vi "FileExplorerMain.vi"(0 "Top Level Folder Path":path, 4 "Tree":string[](tree), 5 "Search Bar":string, 7 "Copy":bool, 9 "Expand / Colapse":bool, 11 "error in (no error)":errorcluster) -> (6 "Report String":string, 15 "error out":errorcluster)   [LabVIEW 2023]
doc: "This VI is the demonstration of the File explorer using tree with options like search, copy, expand/collapse the tree items populated from the input file path."
uses:
  TypeDefs/FileExplorerQueueOperations.ctl
  TypeDefs/FileExplorerStateDataCluster.ctl
  TypeDefs/FileExplorerDataCluster.ctl
  TypeDefs/ReportDetailsCluster.ctl
  TypeDefs/TreeSortCluster.ctl
  TypeDefs/FilesandFoldersPath.ctl
  TypeDefs/FileSelectionCluster.ctl
  TypeDefs/TagsCluster.ctl
panel:
  # "INSTRUCTIONS\n\n1. Run the VI.\n2. Choose the any folder path using \"Top Level Folder Path\" Control.\n3. Tree is populated with the selected folder hierarchy.\n4. Press \"Expand/Collapse\" button to expand or collapse the Folders in the tree.\n5. Enter folder name in the \"Search Bar\" and press enter to expand on particular folder.\n6. Select any files in the tree and press \"Copy\" to copy the file to the desired location.\n7. Whenever a folder is expanded, particular folder details is indicated in the \"Report String\"\n8. Press the Column Headers to sort the tree based on the selection like Date Modified, Type or size"
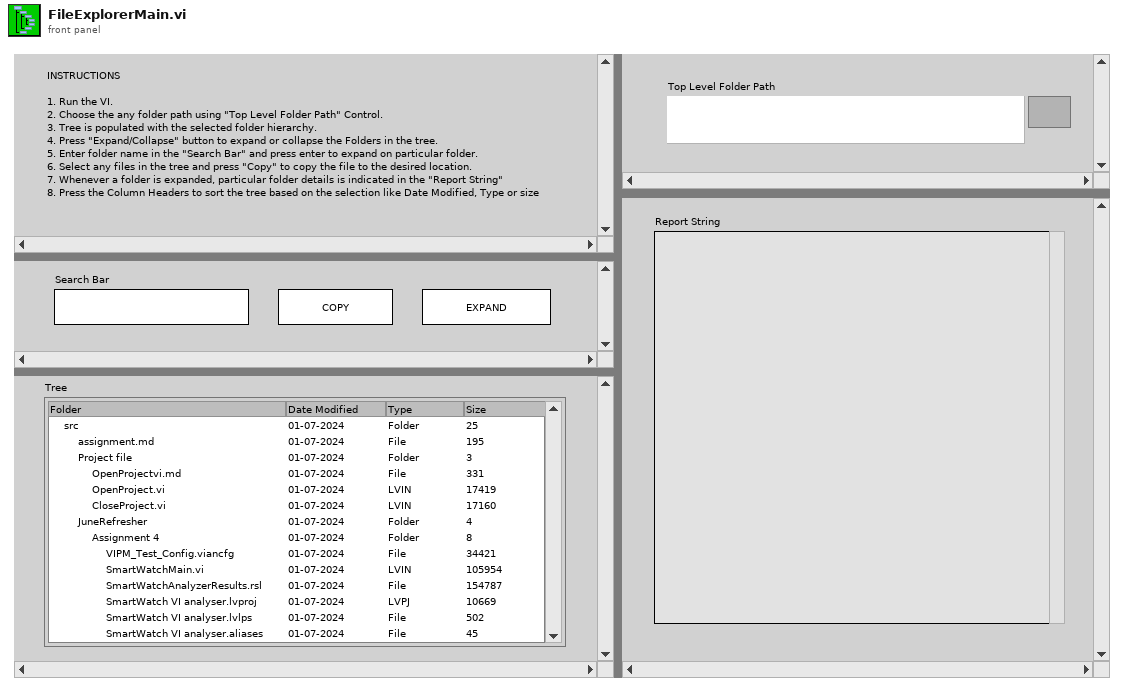
[diagram p1: front panel]
types:
  T1 = typedef "FileExplorerDataCluster.ctl" = cluster{"user event ref":refnum<user-event>, "Search Bar":string, "Tag Path":string[], "Copied File Path array":path[], "Copy file Folder":string, "Folders Array":string[], "Report details":T2, "Sort Flag":T3, "Paths":T4, "File Selection":T5, "Tags":T6, "TagSymbol Array":string[], "Path Tag":string, "New Folder Tag":path, "New Folder":bool, "Folder Found":bool, "Searched Folder Tag":string[]}
  T2 = typedef "ReportDetailsCluster.ctl" = cluster{"Tag Date Modified":string, "Tag Size":string, "Tag Type":string, "Report String":string}
  T3 = typedef "TreeSortCluster.ctl" = cluster{"Sort Date":bool, "Sort Type":bool, "Sort Size":bool}
  T4 = typedef "FilesandFoldersPath.ctl" = cluster{"File Path":path, "All Folders Path":path[], "All Files Path":path[], "Temp File Path":path, "New Folder Dialog":path}
  T5 = typedef "FileSelectionCluster.ctl" = cluster{"Files Selected ?":bool, "Selected file array":string[], "First Selection":string}
  T6 = typedef "TagsCluster.ctl" = cluster{"Parent Tag":string, "Active Tag":string}
  T7 = typedef "FileExplorerStateDataCluster.ctl" = cluster{"State":string, "Data":variant}
  T8 = typedef "FileExplorerQueueOperations.ctl" = enum16{"Init", "Enqueue", "Dequeue", "Enqueue N", "Flush", "Close", "Enqueue N Stack"}
  T9 = typedef "LVPoint32TypeDef.ctl" = cluster{"Horizontal":i32, "Vertical":i32}
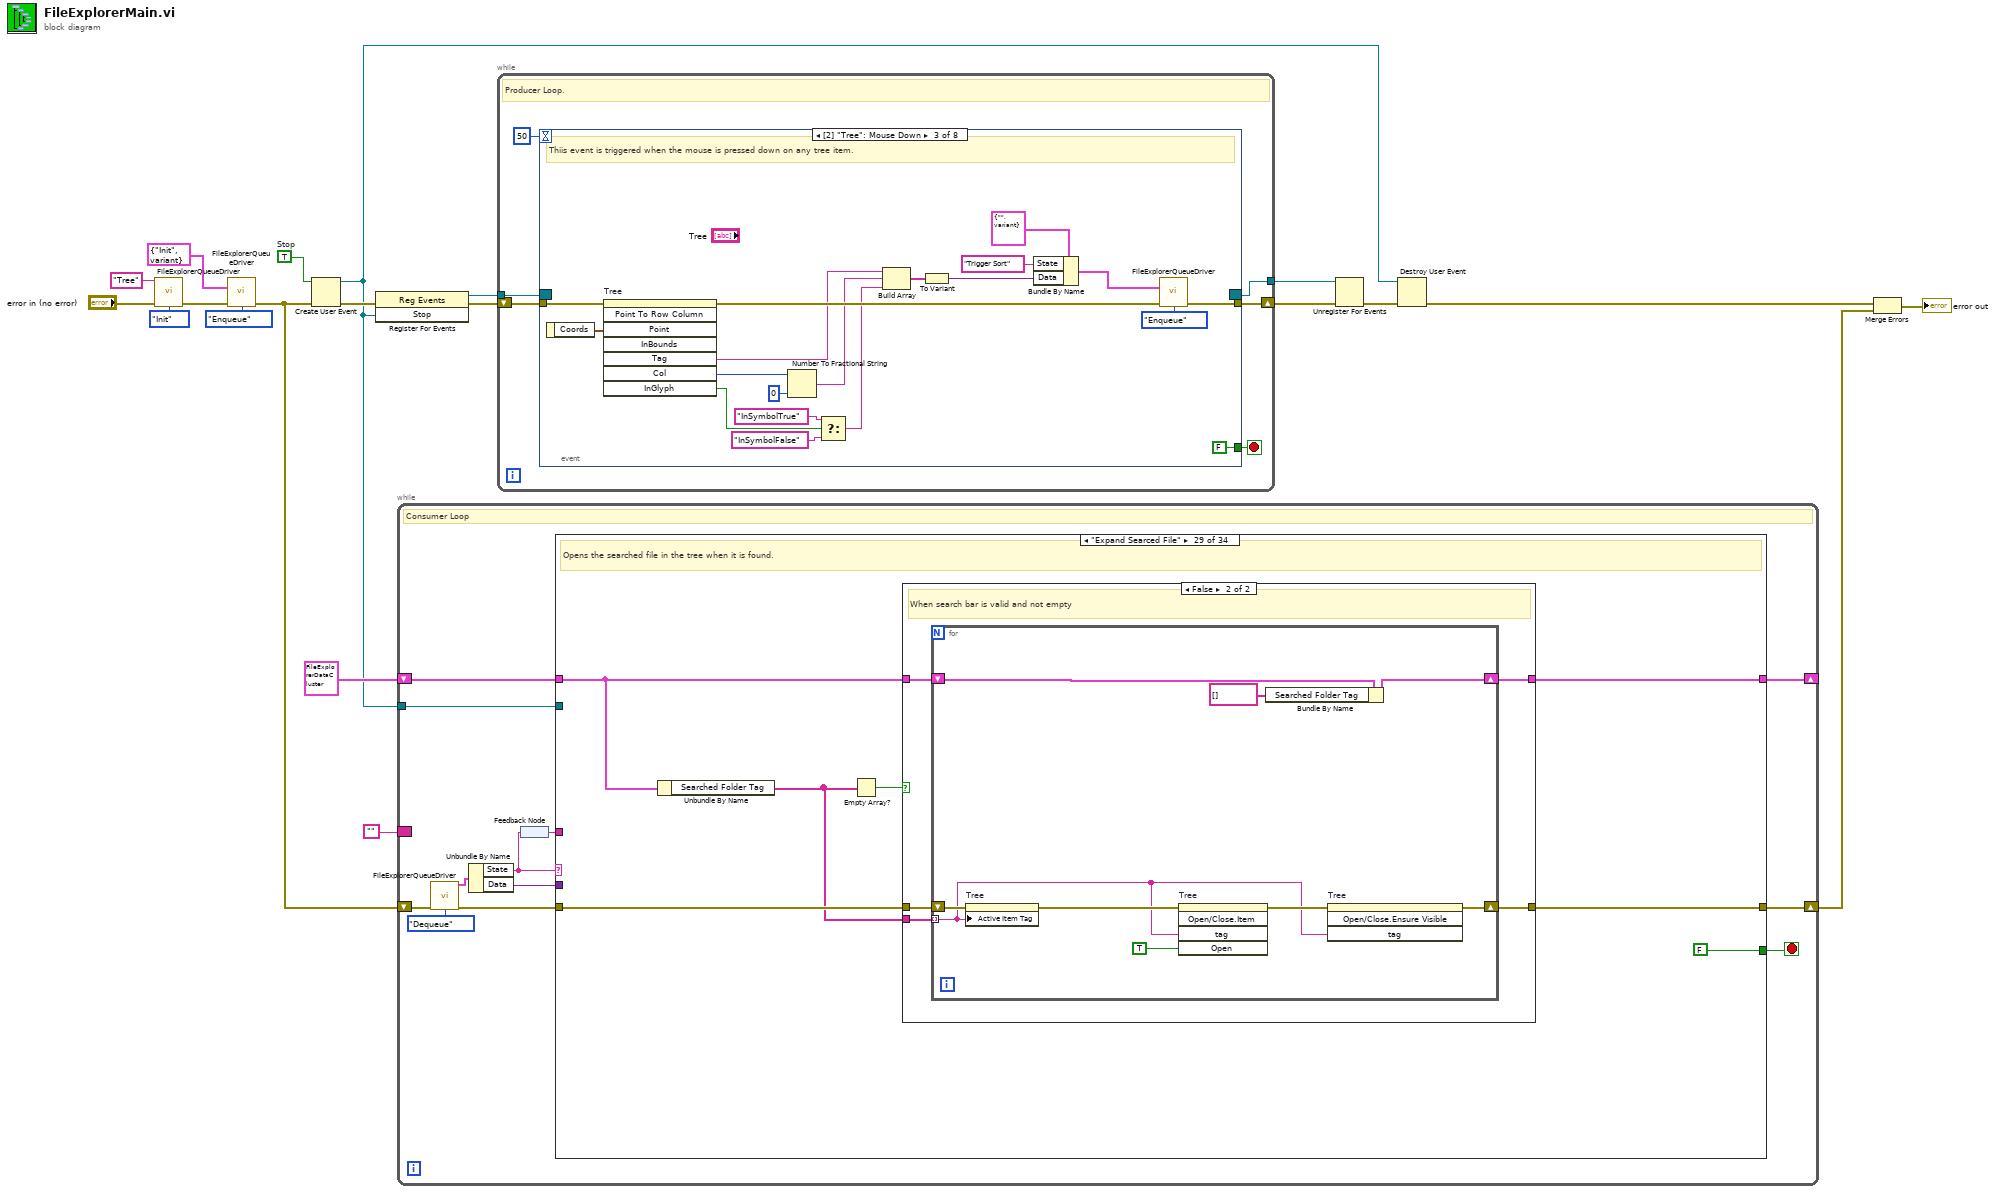
[diagram p0: block diagram]
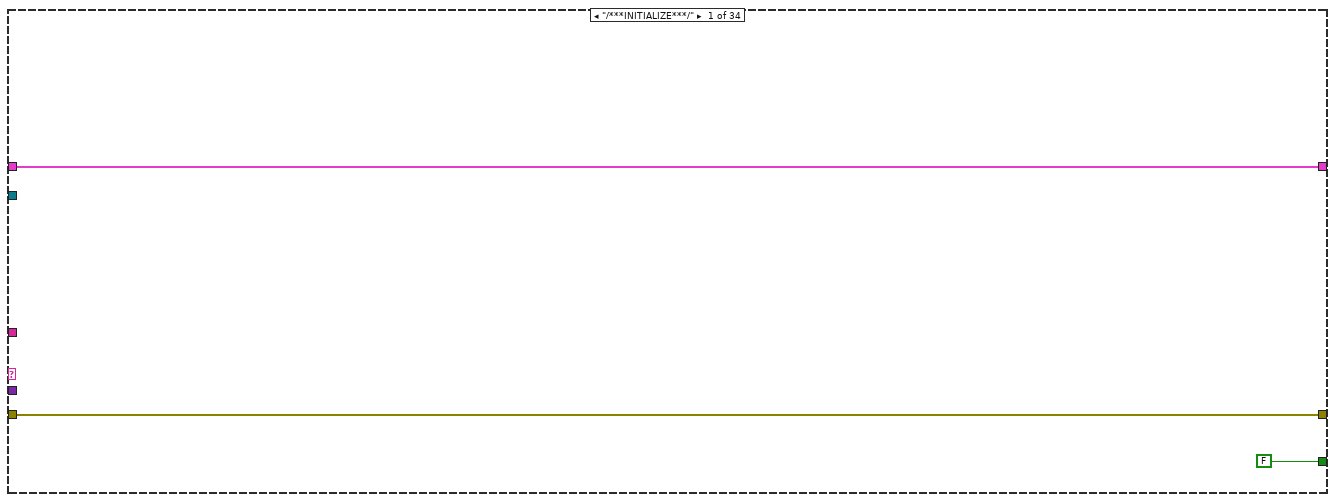
[diagram p2: hidden frame]
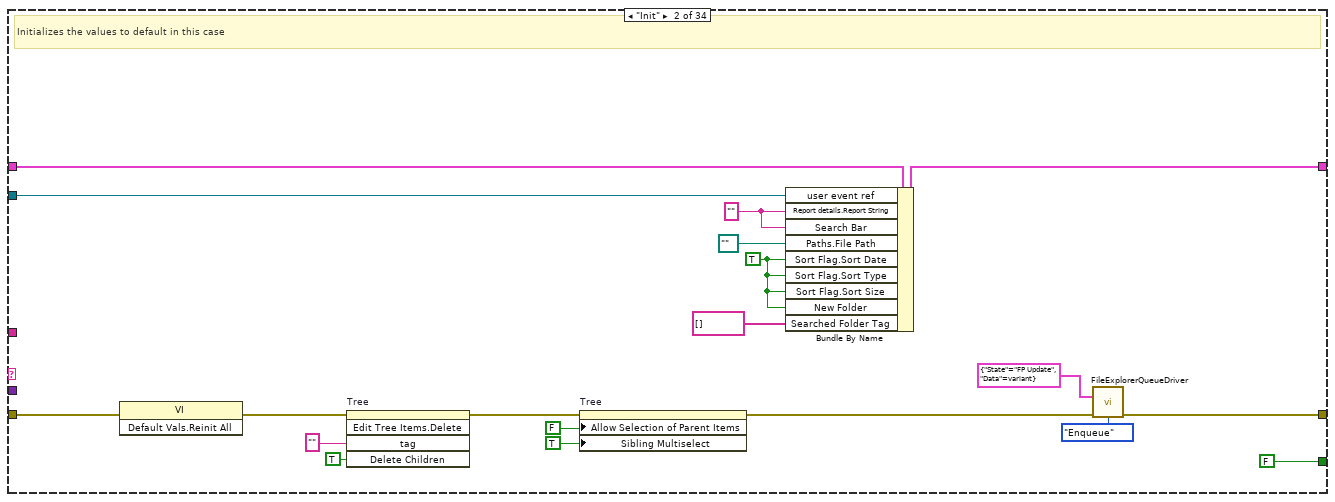
[diagram p3: hidden frame]
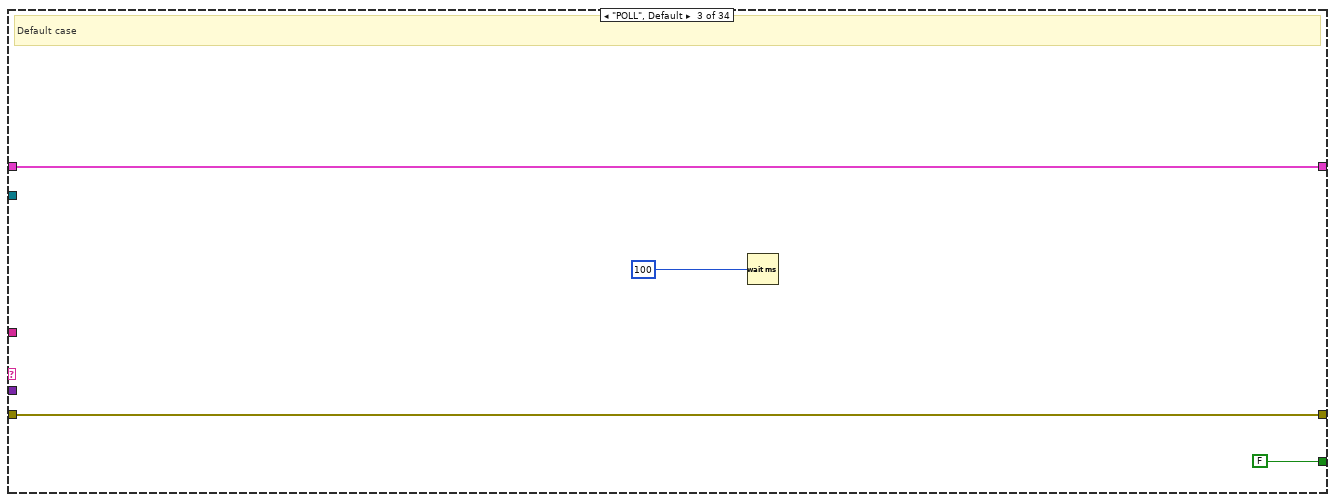
[diagram p4: hidden frame]
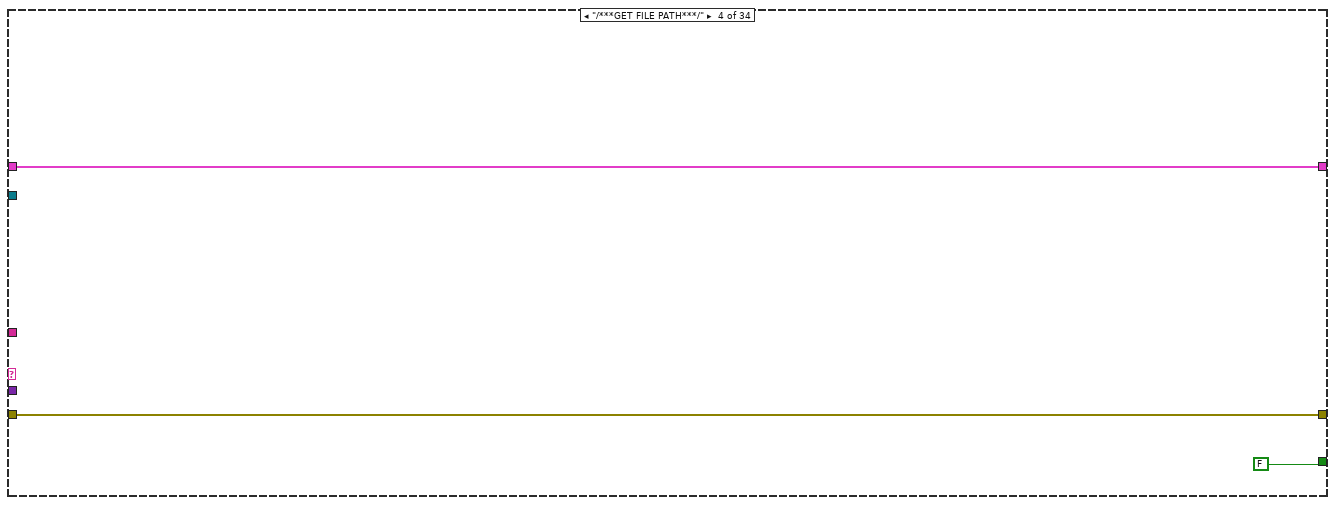
[diagram p5: hidden frame]
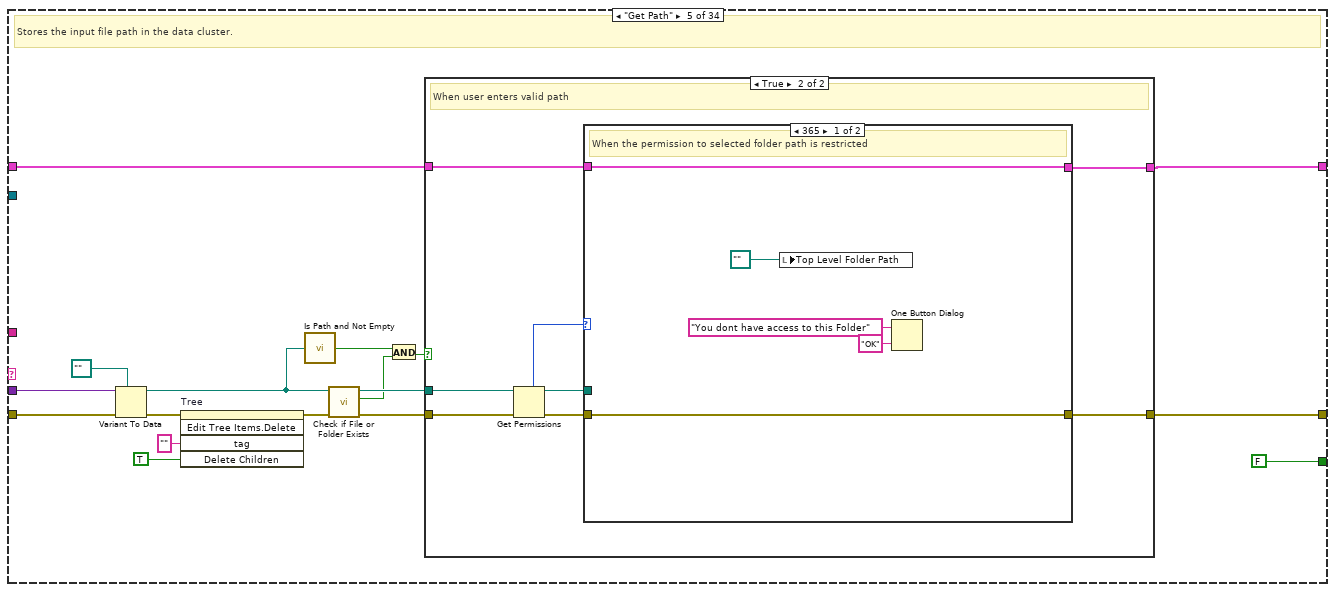
[diagram p6: hidden frame]
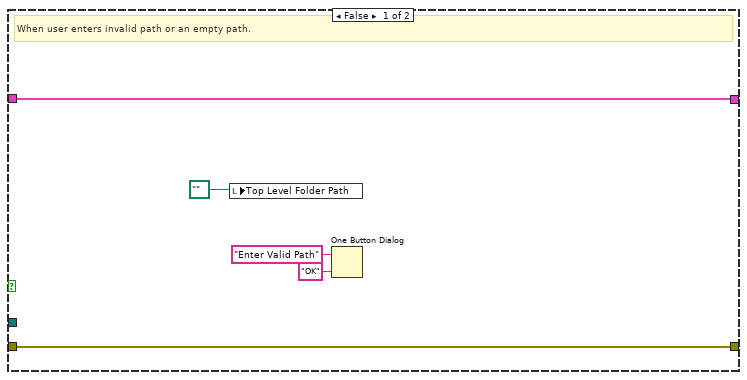
[diagram p7: hidden frame]
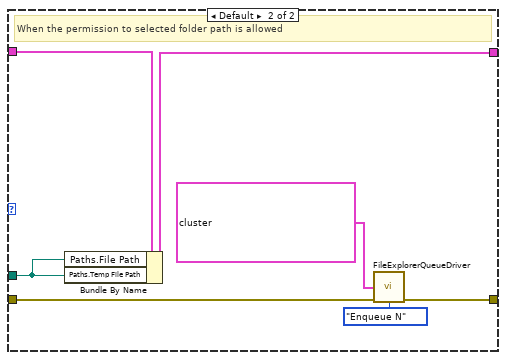
[diagram p8: hidden frame]
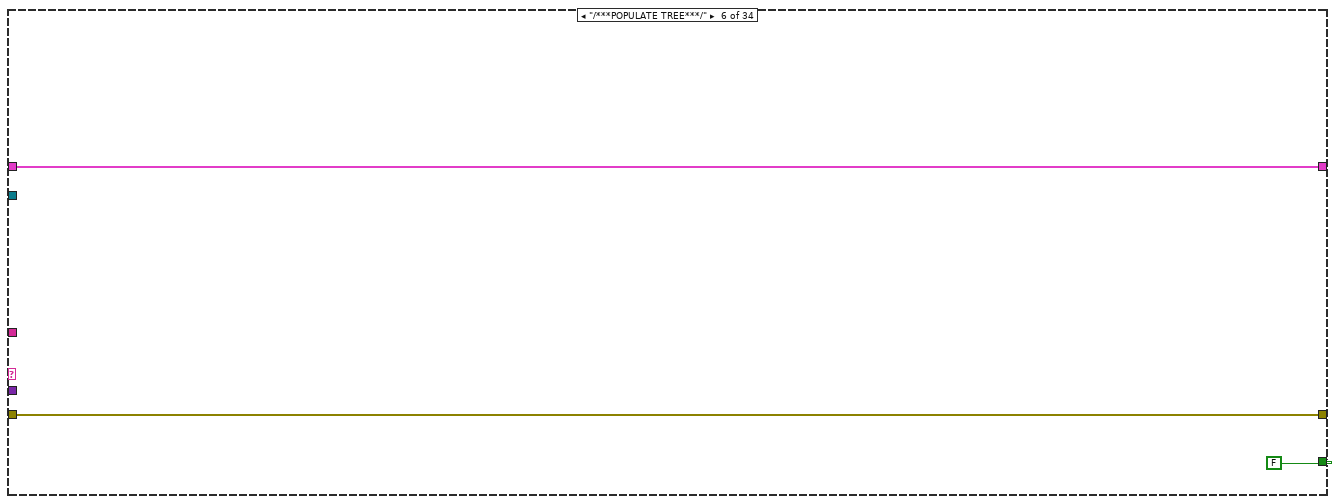
[diagram p9: hidden frame]
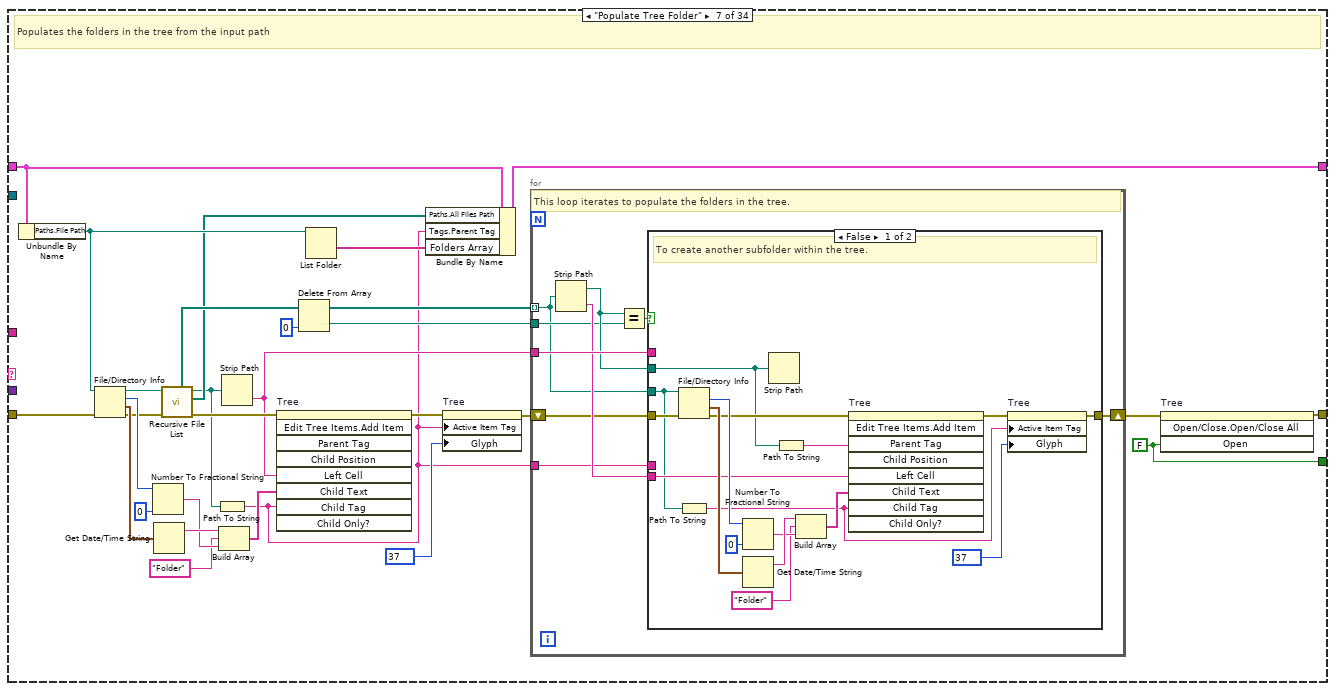
[diagram p10: hidden frame]
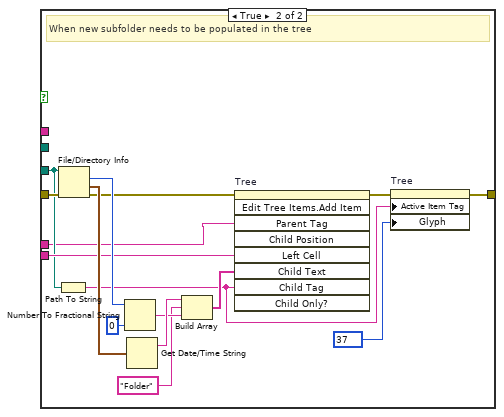
[diagram p11: hidden frame]
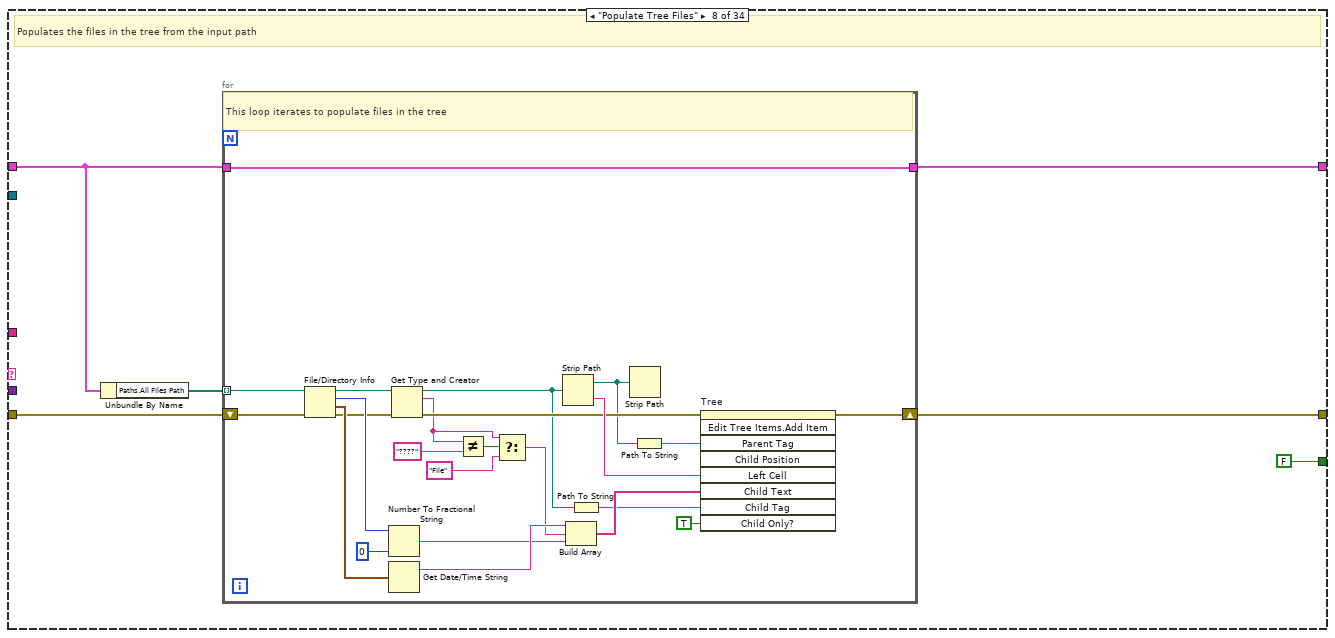
[diagram p12: hidden frame]
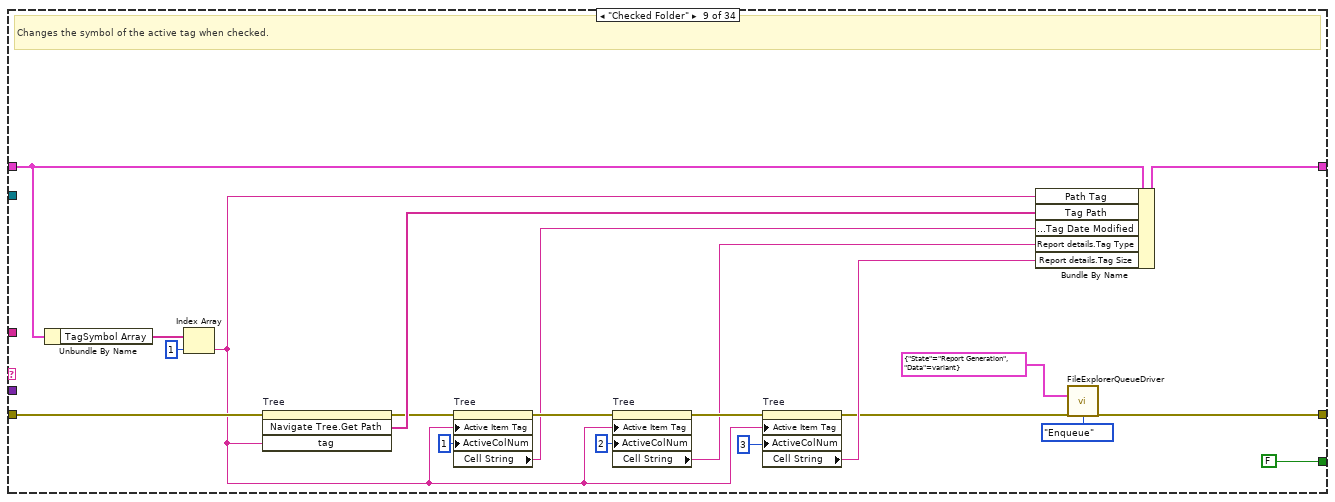
[diagram p13: hidden frame]
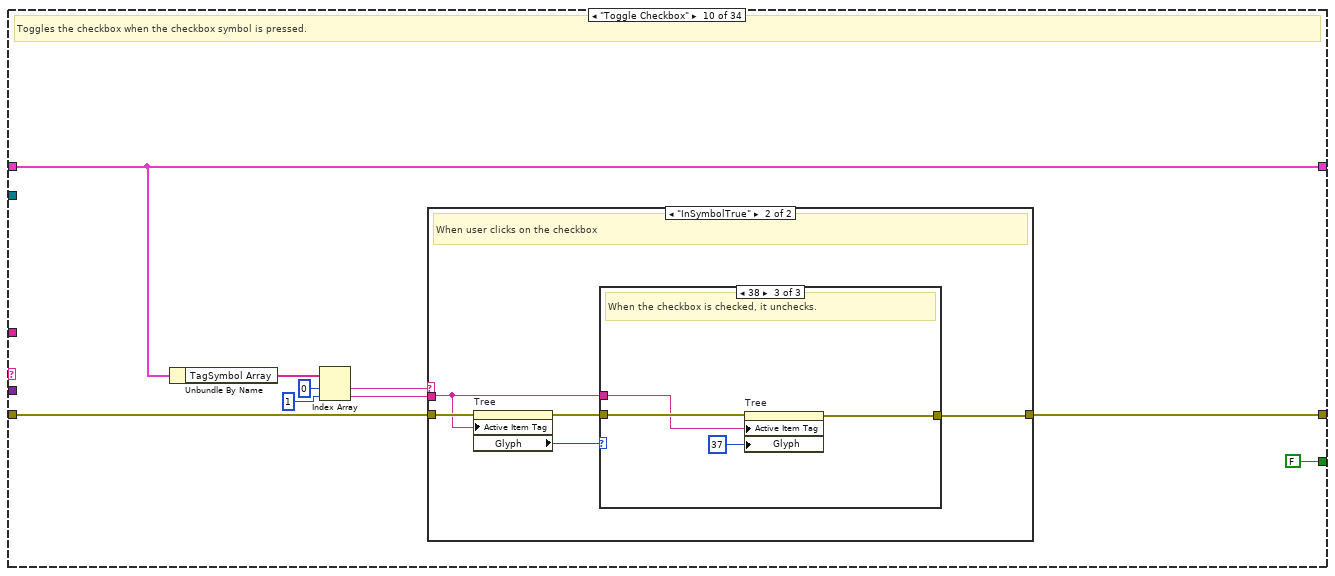
[diagram p14: hidden frame]
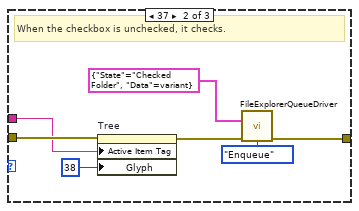
[diagram p17: hidden frame]
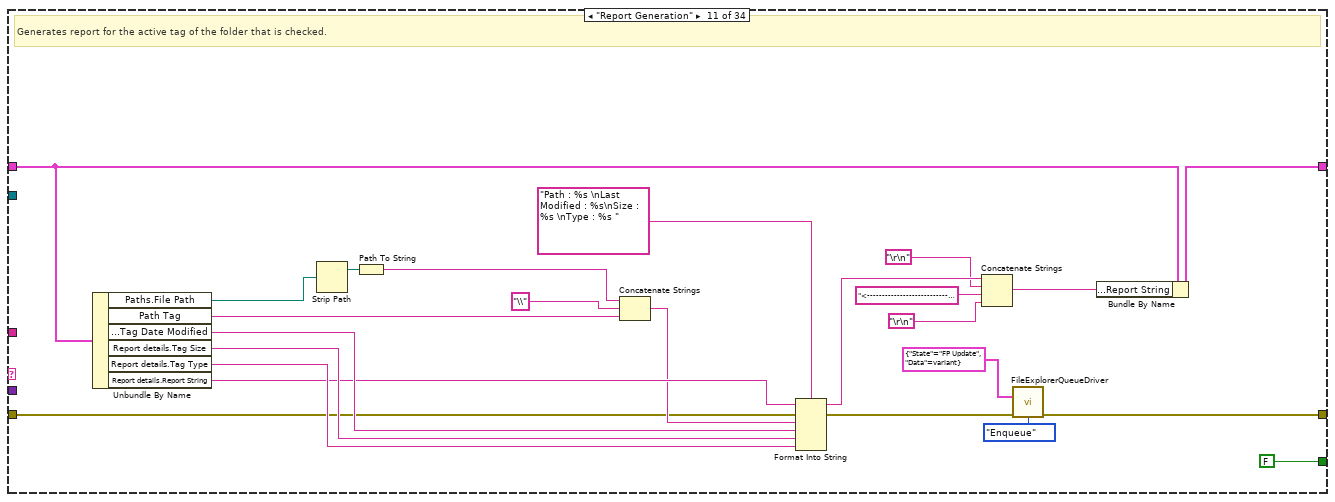
[diagram p18: hidden frame]
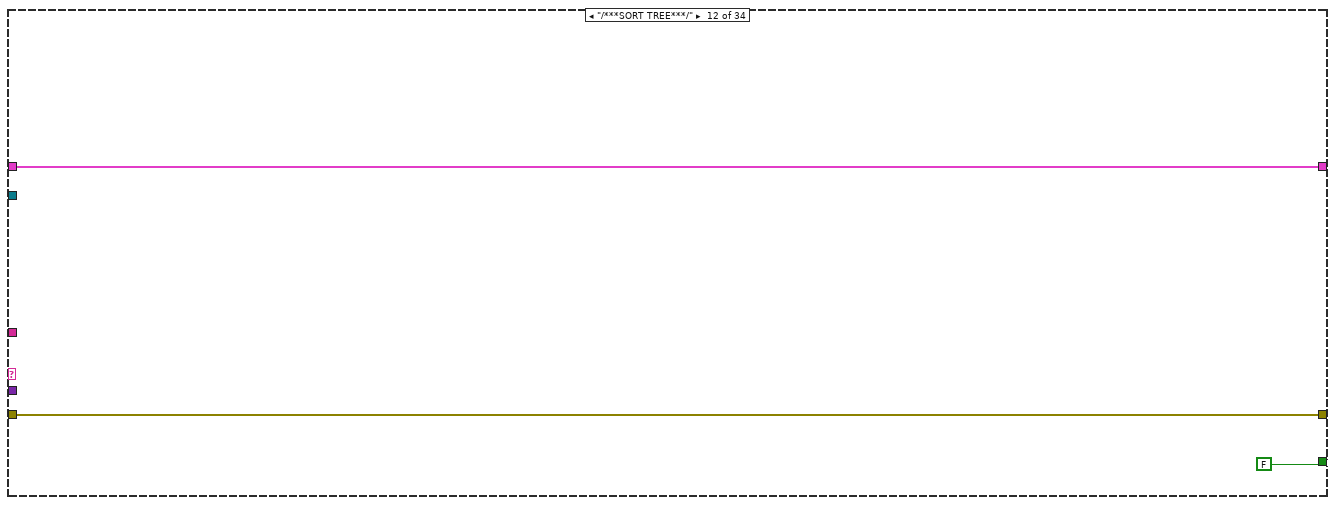
[diagram p19: hidden frame]
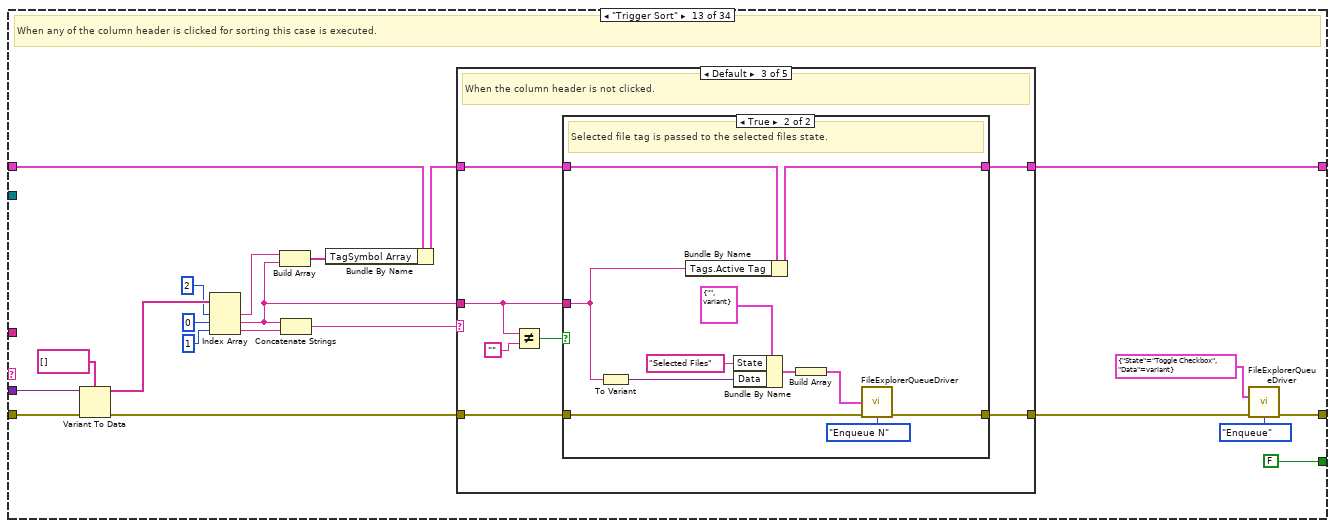
[diagram p20: hidden frame]
diagram:
  w10 = TRUE  # Stop
  n1 = call "FileExplorerQueueDriver.vi"("Queue Name"="Tree", "error in (no error)"="error in (no error)", "Enum"=FileExplorerQueueOperations."Init") -> ("error out"=w13:errorcluster)  [unwired: 11 in, 1 out]
  n2 = call "FileExplorerQueueDriver.vi"("Enqueue Element"=T7 {"State"="Init", "Data"=variant}, "error in (no error)"=w13, "Enum"=FileExplorerQueueOperations."Enqueue") -> ("error out"=w2:errorcluster)  [unwired: 11 in, 1 out]
  n3 = Create User Event(user event datatype=w10, error in=w2) -> (user event=w3:refnum<user-event>, error out=w11:errorcluster)
  n4 = register-events(error in=w11, w3) -> (reference out=w8:refnum<event-registration>, error out=w9:errorcluster)  [unwired: 1 in]
  n5 = while {
    shift-right: [w30] -> w17
    shift-left: w2 -> [w32]
    tunnel: w3 -> [w25]
    shift-right: [w23] -> _
    shift-left: T1 {"user event ref"=refnum, "Search Bar"="", "Tag Path"=[], "Copied File Path array"=[], "Copy file Folder"="", "Folders Array"=[], "Report details"={"Tag Date Modified"="", "Tag Size"="", "Tag Type"="", "Report String"=""}, "Sort Flag"={"Sort Date"=FALSE, "Sort Type"=FALSE, "Sort Size"=FALSE}, "Paths"={"File Path"=path "", "All Folders Path"=[], "All Files Path"=[], "Temp File Path"=path "", "New Folder Dialog"=path ""}, "File Selection"={"Files Selected ?"=FALSE, "Selected file array"=[], "First Selection"=""}, "Tags"={"Parent Tag"="", "Active Tag"=""}, "TagSymbol Array"=[], "Path Tag"="", "New Folder Tag"=path "", "New Folder"=FALSE, "Folder Found"=FALSE, "Searched Folder Tag"=[]} -> [w24]
    border: "" ("State") -> [_]
    stop <- w28 stop-if-true
    # "Consumer Loop"
    n6 = call "FileExplorerQueueDriver.vi"("error in (no error)"=w32, "Enum"=FileExplorerQueueOperations."Dequeue") -> ("Dequeue Element"=w27:T7, "error out"=w31:errorcluster)  [unwired: 12 in]
    n7 = Unbundle By Name(w27) -> ("State"=w22:string, "Data"=w26:variant)
    n8 = feedback #1() -> (w21:string)
    n9 = feedback-in #1(w22) -> ()
    n10 = case shown="\"Expand Searced File\"" w22 {
      tunnel: w31 -> [w34 w48 w58 w60 w76 w105 w114 w181 w212 w232 w257 w281 w303 w350 w380 w415 w426 w432 w458 w463 w513 w540 w590 w628 w678 w690 w700 w715 w736 w760 w765 w767 w780 w801]
      tunnel: [w34 w45 w58 w60 w70 w105 w121 w180 w216 w231 w267 w281 w284 w346 w376 w414 w425 w428 w458 w464 w515 w543 w584 w636 w678 w685 w700 w702 w737 w760 w765 w767 w786 w799] -> w30
      tunnel: [FALSE FALSE FALSE FALSE FALSE FALSE w115 FALSE FALSE FALSE ("Open?") FALSE FALSE FALSE FALSE FALSE FALSE FALSE FALSE FALSE FALSE FALSE ("Open?") FALSE ("Open?") FALSE FALSE FALSE FALSE FALSE FALSE FALSE FALSE FALSE FALSE FALSE TRUE] -> w28
      tunnel: w26 -> [_ _ _ _ w75 _ _ _ _ _ _ _ w302 _ _ w407 w418 _ _ _ _ _ w589 _ _ w688 _ w714 _ _ _ _ _ _]
      tunnel: w25 -> [_ w51 _ _ _ _ _ _ _ _ _ _ _ _ _ _ _ _ _ _ _ _ _ _ _ _ _ _ _ _ _ _ _ _]
      tunnel: w24 -> [w35 w53 w57 w61 w78 w106 w131 w183 w211 w236 w279 w282 w301 w348 w378 w411 w422 w430 w459 w461 w510 w546 w587 w624 w679 w683 w701 w711 w735 w761 w764 w768 w785 w802]
      tunnel: [w35 w52 w57 w61 w77 w106 w130 w178 w228 w236 w271 w282 w300 w347 w377 w411 w422 w429 w459 w465 w509 w546 w586 w635 w679 w681 w701 w710 w738 w761 w764 w768 w783 w802] -> w23
      tunnel: w21 -> [_ _ _ _ _ _ _ _ _ _ _ _ _ _ _ _ _ _ _ _ _ _ _ _ _ _ _ _ _ _ _ _ w777 _]
      frame "/***INITIALIZE***/" {
      }
      frame "Init" {
        w37 = TRUE ("Trigger Sort")
        w47 = "" ("Report String")
        # "Initializes the values to default in this case"
        n11 = invoke class="VI" method="Default Vals.Reinit All"(error in=w48) -> (error out=w43:errorcluster)  [unwired: 2 in, 2 out]
        n12 = invoke on="Tree" class="Tree (strict)" method="Edit Tree Items.Delete"(error in=w43, "tag"="" ("Tag"), "Delete Children"=TRUE ("Delete Children?")) -> (error out=w41:errorcluster)  [unwired: 2 in, 4 out]
        n13 = property on="Tree" class="Tree (strict)"(error in=w41, "Allow Selection of Parent Items"=FALSE ("Sibling Multiselect"), "Sibling Multiselect"=TRUE) -> (error out=w42:errorcluster)  [unwired: 1 in, 1 out]
        n14 = Bundle By Name(cluster=w53, "user event ref"=w51, "Report details.Report String"=w47, "Search Bar"=w47, "Paths.File Path"=path "" ("File Path"), "Sort Flag.Sort Date"=w37, "Sort Flag.Sort Type"=w37, "Sort Flag.Sort Size"=w37, "New Folder"=w37, "Searched Folder Tag"=string[] []) -> (w52:T1)
        n15 = call "FileExplorerQueueDriver.vi"("Enqueue Element"=T7 {"State"="FP Update", "Data"=variant}, "error in (no error)"=w42, "Enum"=FileExplorerQueueOperations."Enqueue") -> ("error out"=w45:errorcluster)  [unwired: 11 in, 1 out]
      }
      frame "POLL", Default {
        # "Default case"
        n16 = Wait (ms)(milliseconds to wait=u32 100) -> ()  [unwired: 1 out]
      }
      frame "/***GET FILE PATH***/" {
      }
      frame "Get Path" {
        # "Stores the input file path in the data cluster."
        n17 = Variant To Data(error in=w76, type=path "" ("NewVal"), Variant=w75) -> (data=w66:path, error out=w72:errorcluster)
        n18 = invoke on="Tree" class="Tree (strict)" method="Edit Tree Items.Delete"(error in=w72, "tag"="" ("Tag"), "Delete Children"=TRUE ("Delete Children?")) -> (error out=w69:errorcluster)  [unwired: 2 in, 4 out]
        n19 = call <vilib>:"Is Path and Not Empty.vi"("path"=w66) -> ("Is Path and Not Empty?"=w63:bool)  [unwired: 4 in]
        n20 = call <vilib>:"Check if File or Folder Exists.vi"("error in (no error)"=w69, "path"=w66) -> ("error out"=w68:errorcluster, "file or folder exists?"=w65:bool, "dup path"=w67:path)  [unwired: 7 in]
        n21 = And(x=w63, y=w65) -> (x .and. y?=w64:bool)
        n22 = case shown="True" w64 {
          tunnel: w78 -> [w83 w91]
          tunnel: [w83 w90] -> w77
          tunnel: w67 -> [_ w87]
          tunnel: w68 -> [w80 w88]
          tunnel: [w80 w89] -> w70
          frame False {
            # "When user enters invalid path or an empty path."
            n23 = local write "Top Level Folder Path"(path "" ("Top Level Folder Path")) -> ()
            n24 = One Button Dialog(message="Enter Valid Path", button name ("OK")="OK") -> ()  [unwired: 1 out]
          }
          frame True {
            # "When user enters valid path"
            n25 = Get Permissions(8:w88, 11:w87) -> (0:w86:errorcluster, 3:w85:path, 5:w84:i16)  [unwired: 2 out]
            n26 = case shown="365" w84 {
              tunnel: w91 -> [w96 w103]
              tunnel: [w96 w102] -> w90
              tunnel: [w93 w100] -> w89
              tunnel: w85 -> [_ w98]
              tunnel: w86 -> [w93 w97]
              frame 365 {
                # "When the permission to selected folder path is restricted"
                n27 = local write "Top Level Folder Path"(path "" ("Top Level Folder Path")) -> ()
                n28 = One Button Dialog(message="You dont have access to this Folder", button name ("OK")="OK") -> ()  [unwired: 1 out]
              }
              frame Default {
                # "When the permission to selected folder path is allowed"
                n29 = Bundle By Name(cluster=w103, "Paths.File Path"=w98, "Paths.Temp File Path"=w98) -> (w102:T1)
                n30 = call "FileExplorerQueueDriver.vi"("Enqueue N Element"=T7[] [{"State"="Populate Tree Folder", "Data"=variant}, {"State"="Populate Tree Files", "Data"=variant}], "error in (no error)"=w97, "Enum"=FileExplorerQueueOperations."Enqueue N") -> ("error out"=w100:errorcluster)  [unwired: 11 in, 1 out]
              }
            }
          }
        }
      }
      frame "/***POPULATE TREE***/" {
      }
      frame "Populate Tree Folder" {
        w115 = FALSE ("Open?")
        # "Populates the folders in the tree from the input path"
        n31 = Unbundle By Name(w131) -> ("Paths.File Path"=w117:path)
        n32 = File/Directory Info(path=w117, error in=w114) -> (path out=w112:path, size=w127:i64, last mod=w129:timestamp, error out=w113:errorcluster)  [unwired: 3 out]
        n33 = Number To Fractional String(number=w127, precision (6)=i16 0) -> (F-format string=w126:string)  [unwired: 2 in]
        n34 = Get Date/Time String(seconds (now)=w129) -> (date string=w128:string)  [unwired: 2 in, 1 out]
        n35 = call <vilib>:"Recursive File List.vi"("error in (no error)"=w113, "Folder Path"=w112) -> ("error out"=w111:errorcluster, "All Files in Dir"=w110:path[], "dup Folder Path"=w109:path, "All Folders"=w134:path[])  [unwired: 5 in, 1 out]
        n36 = Path To String(path=w109) -> (string=w107:string)
        n37 = Build Array(w128, "Folder" ("element"), w126) -> (w123:string[])
        n38 = Strip Path(path=w109) -> (name=w108:string)  [unwired: 1 out]
        n39 = invoke on="Tree" class="Tree (strict)" method="Edit Tree Items.Add Item"(error in=w111, "Left Cell"=w108, "Child Text"=w123, "Child Tag"=w107) -> (error out=w120:errorcluster)  [unwired: 5 in, 8 out]
        n40 = Delete From Array(array=w134, index=0) -> (deleted portion=w132:path, array with subset deleted=w133:path[])  [unwired: 1 in]
        n41 = List Folder(path=w117) -> (folder names=w116:string[])  [unwired: 3 in, 3 out]
        n42 = Bundle By Name(cluster=w131, "Paths.All Files Path"=w110, "Tags.Parent Tag"=w107, "Folders Array"=w116) -> (w130:T1)
        n43 = property on="Tree" class="Tree (strict)"(error in=w120, "Active Item Tag"=w107, "Glyph"=37) -> (error out=w119:errorcluster)  [unwired: 1 in, 1 out]
        n44 = for {
          tunnel: w133 -> [w137] mode=indexing
          tunnel: w108 -> [w144]
          tunnel: w132 -> [w138]
          shift-right: [w139] -> w122
          shift-left: w119 -> [w140]
          tunnel: w107 -> [w136]
          # "This loop iterates to populate the folders in the tree."
          n45 = Strip Path(path=w137) -> (stripped path=w141:path, name=w143:string)
          n46 = Equal?(x=w141, y=w138) -> (x = y?=w142:bool)
          n47 = case shown="False" w142 {
            tunnel: w144 -> [_ _]
            tunnel: w143 -> [w151 w168]
            tunnel: w141 -> [w146 _]
            tunnel: w140 -> [w150 w166]
            tunnel: [w152 w169] -> w139
            tunnel: w137 -> [w148 w164]
            tunnel: w136 -> [_ w162]
            frame False {
              # "To create another subfolder within the tree."
              n48 = File/Directory Info(path=w148, error in=w150) -> (size=w159:i64, last mod=w161:timestamp, error out=w149:errorcluster)  [unwired: 4 out]
              n49 = Path To String(path=w148) -> (string=w147:string)
              n50 = Number To Fractional String(number=w159, precision (6)=i16 0) -> (F-format string=w158:string)  [unwired: 2 in]
              n51 = Get Date/Time String(seconds (now)=w161) -> (date string=w160:string)  [unwired: 2 in, 1 out]
              n52 = Strip Path(path=w146) -> ()  [unwired: 2 out]
              n53 = Path To String(path=w146) -> (string=w145:string)
              n54 = Build Array(w160, "Folder" ("element"), w158) -> (w156:string[])
              n55 = invoke on="Tree" class="Tree (strict)" method="Edit Tree Items.Add Item"(error in=w149, "Parent Tag"=w145, "Left Cell"=w151, "Child Text"=w156, "Child Tag"=w147) -> (error out=w153:errorcluster)  [unwired: 4 in, 8 out]
              n56 = property on="Tree" class="Tree (strict)"(error in=w153, "Active Item Tag"=w147, "Glyph"=37 ("Active Item:Symbol Index")) -> (error out=w152:errorcluster)  [unwired: 1 in, 1 out]
            }
            frame True {
              # "When new subfolder needs to be populated in the tree"
              n57 = Path To String(path=w164) -> (string=w163:string)
              n58 = File/Directory Info(path=w164, error in=w166) -> (size=w175:i64, last mod=w177:timestamp, error out=w165:errorcluster)  [unwired: 4 out]
              n59 = Number To Fractional String(number=w175, precision (6)=i16 0) -> (F-format string=w174:string)  [unwired: 2 in]
              n60 = Get Date/Time String(seconds (now)=w177) -> (date string=w176:string)  [unwired: 2 in, 1 out]
              n61 = Build Array(w176, "Folder" ("element"), w174) -> (w172:string[])
              n62 = invoke on="Tree" class="Tree (strict)" method="Edit Tree Items.Add Item"(error in=w165, "Parent Tag"=w162, "Left Cell"=w168, "Child Text"=w172, "Child Tag"=w163) -> (error out=w170:errorcluster)  [unwired: 4 in, 8 out]
              n63 = property on="Tree" class="Tree (strict)"(error in=w170, "Active Item Tag"=w163, "Glyph"=37) -> (error out=w169:errorcluster)  [unwired: 1 in, 1 out]
            }
          }
        }
        n64 = invoke on="Tree" class="Tree (strict)" method="Open/Close.Open/Close All"(error in=w122, "Open"=w115) -> (error out=w121:errorcluster)  [unwired: 2 in, 3 out]
      }
      frame "Populate Tree Files" {
        # "Populates the files in the tree from the input path"
        n65 = Unbundle By Name(w183) -> ("Paths.All Files Path"=w182:path[])
        n66 = for {
          tunnel: w183 -> [w207]
          tunnel: [w207] -> w178
          tunnel: w182 -> [w203] mode=indexing
          shift-right: [w206] -> w180
          shift-left: w181 -> [w196]
          # "This loop iterates to populate files in the tree"
          n67 = File/Directory Info(path=w203, error in=w196) -> (path out=w194:path, size=w202:i64, last mod=w205:timestamp, error out=w195:errorcluster)  [unwired: 3 out]
          n68 = Number To Fractional String(number=w202, precision (6)=i16 0) -> (F-format string=w201:string)  [unwired: 2 in]
          n69 = Get Date/Time String(seconds (now)=w205) -> (date string=w204:string)  [unwired: 2 in, 1 out]
          n70 = Get Type and Creator(4:w195, 7:w194) -> (0:w193:errorcluster, 2:w190:string, 3:w187:path)  [unwired: 1 out]
          n71 = Not Equal?(x=w190, y="????") -> (x != y?=w191:bool)
          n72 = Select(t=w190, s=w191, f="File") -> (s? t:f=w188:string)
          n73 = Strip Path(path=w187) -> (stripped path=w185:path, name=w198:string)
          n74 = Build Array(w204, w188, w201) -> (w200:string[])
          n75 = Path To String(path=w187) -> (string=w186:string)
          n76 = Strip Path(path=w185) -> ()  [unwired: 2 out]
          n77 = Path To String(path=w185) -> (string=w184:string)
          n78 = invoke on="Tree" class="Tree (strict)" method="Edit Tree Items.Add Item"(error in=w193, "Parent Tag"=w184, "Left Cell"=w198, "Child Text"=w200, "Child Tag"=w186, "Child Only?"=TRUE) -> (error out=w206:errorcluster)  [unwired: 3 in, 8 out]
        }
      }
      frame "Checked Folder" {
        # "Changes the symbol of the active tag when checked."
        n79 = Unbundle By Name(w211) -> ("TagSymbol Array"=w210:string[])
        n80 = Index Array(array=w210, index=1) -> (element=w208:string)
        n81 = invoke on="Tree" class="Tree (strict)" method="Navigate Tree.Get Path"(error in=w212, "tag"=w208) -> (error out=w223:errorcluster, "Navigate Tree:Get Path"=w227:string[])  [unwired: 2 in, 2 out]
        n82 = property on="Tree" class="Tree (strict)"(error in=w223, "Active Item Tag"=w208, "ActiveColNum"=1 ("Active Cell:Active Column Number")) -> (error out=w224:errorcluster, "Cell String"=w220:string)  [unwired: 1 in, 1 out]
        n83 = property on="Tree" class="Tree (strict)"(error in=w224, "Active Item Tag"=w208, "ActiveColNum"=2 ("Active Cell:Active Column Number")) -> (error out=w225:errorcluster, "Cell String"=w219:string)  [unwired: 1 in, 1 out]
        n84 = property on="Tree" class="Tree (strict)"(error in=w225, "Active Item Tag"=w208, "ActiveColNum"=3 ("Active Cell:Active Column Number")) -> (error out=w214:errorcluster, "Cell String"=w218:string)  [unwired: 1 in, 1 out]
        n85 = Bundle By Name(cluster=w211, "Path Tag"=w208, "Tag Path"=w227, "Report details.Tag Date Modified"=w220, "Report details.Tag Type"=w219, "Report details.Tag Size"=w218) -> (w228:T1)
        n86 = call "FileExplorerQueueDriver.vi"("Enqueue Element"=T7 {"State"="Report Generation", "Data"=variant}, "error in (no error)"=w214, "Enum"=FileExplorerQueueOperations."Enqueue") -> ("error out"=w216:errorcluster)  [unwired: 11 in, 1 out]
      }
      frame "Toggle Checkbox" {
        # "Toggles the checkbox when the checkbox symbol is pressed."
        n87 = Unbundle By Name(w236) -> ("TagSymbol Array"=w235:string[])
        n88 = Index Array(array=w235, index #1=0 ("index"), index #2=1 ("index")) -> (element #1=w230:string, element #2=w229:string)
        n89 = case shown="\"InSymbolTrue\"" w230 {
          tunnel: w232 -> [w238 w243]
          tunnel: [w238 w241] -> w231
          tunnel: w229 -> [_ w239]
          frame "False", Default {
            # "Default case."
          }
          frame "InSymbolTrue" {
            # "When user clicks on the checkbox"
            n90 = property on="Tree" class="Tree (strict)"(error in=w243, "Active Item Tag"=w239) -> (error out=w242:errorcluster, "Glyph"=w240:i32)  [unwired: 1 in, 1 out]
            n91 = case shown="38" w240 {
              tunnel: w242 -> [w244 w251 w255]
              tunnel: [w244 w247 w254] -> w241
              tunnel: w239 -> [_ w250 w253]
              frame Default {
                # "Default case."
              }
              frame 37 {
                # "When the checkbox is unchecked, it checks."
                n92 = property on="Tree" class="Tree (strict)"(error in=w251, "Active Item Tag"=w250, "Glyph"=38 ("Active Item:Symbol Index")) -> (error out=w248:errorcluster)  [unwired: 1 in, 1 out]
                n93 = call "FileExplorerQueueDriver.vi"("Enqueue Element"=T7 {"State"="Checked Folder", "Data"=variant}, "error in (no error)"=w248, "Enum"=FileExplorerQueueOperations."Enqueue") -> ("error out"=w247:errorcluster)  [unwired: 11 in, 1 out]
              }
              frame 38 {
                # "When the checkbox is checked, it unchecks."
                n94 = property on="Tree" class="Tree (strict)"(error in=w255, "Active Item Tag"=w253, "Glyph"=37 ("Active Item:Symbol Index")) -> (error out=w254:errorcluster)  [unwired: 1 in, 1 out]
              }
            }
          }
        }
      }
      frame "Report Generation" {
        # "Generates report for the active tag of the folder that is checked."
        n95 = Unbundle By Name(w279) -> ("Paths.File Path"=w261:path, "Path Tag"=w273:string, "Report details.Tag Date Modified"=w277:string, "Report details.Tag Size"=w276:string, "Report details.Tag Type"=w275:string, "Report details.Report String"=w274:string)
        n96 = Strip Path(path=w261) -> (stripped path=w259:path)  [unwired: 1 out]
        n97 = Path To String(path=w259) -> (string=w272:string)
        n98 = Concatenate Strings(w272, "\\" ("string"), w273) -> (w260:string)
        n99 = Format Into String(format string="Path : %s \nLast Modified : %s\nSize : %s \nType : %s ", initial string=w274, error in=w257, w260, w277, w276, w275) -> (resulting string=w270:string, error out=w268:errorcluster)
        n100 = Concatenate Strings(w270, "\r\n", "<---------------------------------------------->" ("string"), "\r\n") -> (w265:string)
        n101 = call "FileExplorerQueueDriver.vi"("Enqueue Element"=T7 {"State"="FP Update", "Data"=variant}, "error in (no error)"=w268, "Enum"=FileExplorerQueueOperations."Enqueue") -> ("error out"=w267:errorcluster)  [unwired: 11 in, 1 out]
        n102 = Bundle By Name(cluster=w279, "Report details.Report String"=w265) -> (w271:T1)
      }
      frame "/***SORT TREE***/" {
      }
      frame "Trigger Sort" {
        # "When any of the column header is clicked for sorting this case is executed."
        n103 = Variant To Data(error in=w303, type=string[] [] ("appended array"), Variant=w302) -> (data=w298:string[], error out=w299:errorcluster)
        n104 = Index Array(array=w298, index #1=2 ("index"), index #2=0 ("index"), index #3=1 ("index")) -> (element #1=w289:string, element #2=w288:string, element #3=w294:string)
        n105 = Build Array(w289, w288) -> (w287:string[])
        n106 = Concatenate Strings(w288, w294) -> (w293:string)
        n107 = Bundle By Name(cluster=w301, "TagSymbol Array"=w287) -> (w290:T1)
        n108 = case shown="Default" w293 {
          tunnel: w290 -> [w308 w312 w319 w339 w344]
          tunnel: [w308 w312 w316 w339 w344] -> w300
          tunnel: w299 -> [w306 w311 w318 w337 w342]
          tunnel: [w305 w311 w317 w336 w341] -> w285
          tunnel: w288 -> [_ _ w314 _ _]
          frame "TREE_COLUMN_HEADERS1" {
            # "When Date modified is clicked to sort the tree."
            n109 = call "FileExplorerQueueDriver.vi"("Enqueue Element"=T7 {"State"="Sort by Date Modified", "Data"=variant}, "error in (no error)"=w306, "Enum"=FileExplorerQueueOperations."Enqueue") -> ("error out"=w305:errorcluster)  [unwired: 11 in, 1 out]
          }
          frame "TREE_COLUMN_HEADERS0" {
            # "Click on the main header is considered as invalid selection"
            n110 = One Button Dialog(message="Invalid Selection", button name ("OK")="OK") -> ()  [unwired: 1 out]
          }
          frame Default {
            # "When the column header is not clicked."
            n111 = Not Equal?(x=w314, y="") -> (x != y?=w313:bool)
            n112 = case shown="True" w313 {
              tunnel: w319 -> [w323 w334]
              tunnel: w318 -> [w322 w327]
              tunnel: [w322 w326] -> w317
              tunnel: [w323 w325] -> w316
              tunnel: w314 -> [_ w324]
              frame False {
                # "When there is an invalid selection of tree item"
                n113 = One Button Dialog(message="Invalid Selection", button name ("OK")="OK") -> ()  [unwired: 1 out]
              }
              frame True {
                # "Selected file tag is passed to the selected files state."
                n114 = To Variant(anything=w324) -> (Variant=w328:variant)
                n115 = Bundle By Name(cluster=w334, "Tags.Active Tag"=w324) -> (w325:T1)
                n116 = Bundle By Name(cluster=T7 {"State"="", "Data"=variant} ("Dequeue Element"), "State"="Selected Files", "Data"=w328) -> (w330:T7)
                n117 = Build Array(w330) -> (w329:T7[])
                n118 = call "FileExplorerQueueDriver.vi"("Enqueue N Element"=w329, "error in (no error)"=w327, "Enum"=FileExplorerQueueOperations."Enqueue N") -> ("error out"=w326:errorcluster)  [unwired: 11 in, 1 out]
              }
            }
          }
          frame "TREE_COLUMN_HEADERS3" {
            # "When size is clicked to sort the tree."
            n119 = call "FileExplorerQueueDriver.vi"("Enqueue Element"=T7 {"State"="Sort by Size", "Data"=variant}, "error in (no error)"=w337, "Enum"=FileExplorerQueueOperations."Enqueue") -> ("error out"=w336:errorcluster)  [unwired: 11 in, 1 out]
          }
          frame "TREE_COLUMN_HEADERS2" {
            # "When Type is clicked to sort the tree."
            n120 = call "FileExplorerQueueDriver.vi"("Enqueue Element"=T7 {"State"="Sort by Type", "Data"=variant}, "error in (no error)"=w342, "Enum"=FileExplorerQueueOperations."Enqueue") -> ("error out"=w341:errorcluster)  [unwired: 11 in, 1 out]
          }
        }
        n121 = call "FileExplorerQueueDriver.vi"("Enqueue Element"=T7 {"State"="Toggle Checkbox", "Data"=variant}, "error in (no error)"=w285, "Enum"=FileExplorerQueueOperations."Enqueue") -> ("error out"=w284:errorcluster)  [unwired: 11 in, 1 out]
      }
      frame "Sort by Date Modified" {
        # "When Date modified header is clicked the tree is sorted by the date modified."
        n122 = Unbundle By Name(w348) -> ("Sort Flag.Sort Date"=w349:bool)
        n123 = case shown="True" w349 {
          tunnel: w348 -> [w362 w374]
          tunnel: [w361 w373] -> w347
          tunnel: w350 -> [w354 w366]
          tunnel: [w353 w365] -> w346
          frame False {
            # "When Date modified is clicked for the second time"
            n124 = To Variant(anything=1) -> (Variant=w351:variant)
            n125 = Bundle By Name(cluster=T7 {"State"="", "Data"=variant} ("Dequeue Element"), "State"="Sort Tree Descending", "Data"=w351) -> (w356:T7)
            n126 = Bundle By Name(cluster=w362, "Sort Flag.Sort Date"=TRUE ("Trigger Sort")) -> (w361:T1)
            n127 = Build Array(w356) -> (w355:T7[])
            n128 = call "FileExplorerQueueDriver.vi"("Enqueue N Element"=w355, "error in (no error)"=w354, "Enum"=FileExplorerQueueOperations."Enqueue N") -> ("error out"=w353:errorcluster)  [unwired: 11 in, 1 out]
          }
          frame True {
            # "When Date modified is clicked once"
            n129 = To Variant(anything=1) -> (Variant=w363:variant)
            n130 = Bundle By Name(cluster=T7 {"State"="", "Data"=variant} ("Dequeue Element"), "State"="Sort Tree Ascending", "Data"=w363) -> (w368:T7)
            n131 = Bundle By Name(cluster=w374, "Sort Flag.Sort Date"=FALSE ("Trigger Sort")) -> (w373:T1)
            n132 = Build Array(w368) -> (w367:T7[])
            n133 = call "FileExplorerQueueDriver.vi"("Enqueue N Element"=w367, "error in (no error)"=w366, "Enum"=FileExplorerQueueOperations."Enqueue N") -> ("error out"=w365:errorcluster)  [unwired: 11 in, 1 out]
          }
        }
      }
      frame "Sort by Type" {
        # "When Type header is clicked the tree is sorted by the Type order."
        n134 = Unbundle By Name(w378) -> ("Sort Flag.Sort Type"=w379:bool)
        n135 = case shown="True" w379 {
          tunnel: w378 -> [w392 w404]
          tunnel: [w391 w403] -> w377
          tunnel: w380 -> [w384 w396]
          tunnel: [w383 w395] -> w376
          frame False {
            # "When Type is clicked for the second time"
            n136 = To Variant(anything=2) -> (Variant=w381:variant)
            n137 = Bundle By Name(cluster=T7 {"State"="", "Data"=variant} ("Dequeue Element"), "State"="Sort Tree Descending", "Data"=w381) -> (w386:T7)
            n138 = Bundle By Name(cluster=w392, "Sort Flag.Sort Type"=TRUE ("Trigger Sort")) -> (w391:T1)
            n139 = Build Array(w386) -> (w385:T7[])
            n140 = call "FileExplorerQueueDriver.vi"("Enqueue N Element"=w385, "error in (no error)"=w384, "Enum"=FileExplorerQueueOperations."Enqueue N") -> ("error out"=w383:errorcluster)  [unwired: 11 in, 1 out]
          }
          frame True {
            # "When type is clicked for the second time"
            n141 = To Variant(anything=2) -> (Variant=w393:variant)
            n142 = Bundle By Name(cluster=T7 {"State"="", "Data"=variant} ("Dequeue Element"), "State"="Sort Tree Ascending", "Data"=w393) -> (w398:T7)
            n143 = Bundle By Name(cluster=w404, "Sort Flag.Sort Type"=FALSE ("Trigger Sort")) -> (w403:T1)
            n144 = Build Array(w398) -> (w397:T7[])
            n145 = call "FileExplorerQueueDriver.vi"("Enqueue N Element"=w397, "error in (no error)"=w396, "Enum"=FileExplorerQueueOperations."Enqueue N") -> ("error out"=w395:errorcluster)  [unwired: 11 in, 1 out]
          }
        }
      }
      frame "Sort Tree Ascending" {
        # "Sorts the tree in ascending order when clicked once"
        n146 = Variant To Data(error in=w415, type=1 ("Sort Column"), Variant=w407) -> (data=w406:i32, error out=w409:errorcluster)
        n147 = Unbundle By Name(w411) -> ("Tags.Parent Tag"=w410:string)
        n148 = invoke on="Tree" class="Tree (strict)" method="Edit Tree Items.Sort Children"(error in=w409, "tag"=w410, "Sort Column"=w406, "Sort Recursively"=TRUE ("Sort Recursively?"), "Reverse Order"=FALSE ("Reverse Order?")) -> (error out=w414:errorcluster)  [unwired: 3 in, 7 out]
      }
      frame "Sort Tree Descending" {
        # "Sorts the tree in descending order when clicked for the second time."
        n149 = Variant To Data(error in=w426, type=1 ("Sort Column"), Variant=w418) -> (data=w417:i32, error out=w420:errorcluster)
        n150 = Unbundle By Name(w422) -> ("Tags.Parent Tag"=w421:string)
        n151 = invoke on="Tree" class="Tree (strict)" method="Edit Tree Items.Sort Children"(error in=w420, "tag"=w421, "Sort Column"=w417, "Sort Recursively"=TRUE ("Sort Recursively?"), "Reverse Order"=TRUE ("Reverse Order?")) -> (error out=w425:errorcluster)  [unwired: 3 in, 7 out]
      }
      frame "Sort by Size" {
        # "When Size header is clicked the tree is sorted according to the size."
        n152 = Unbundle By Name(w430) -> ("Sort Flag.Sort Size"=w431:bool)
        n153 = case shown="False" w431 {
          tunnel: w430 -> [w444 w456]
          tunnel: [w443 w455] -> w429
          tunnel: w432 -> [w436 w448]
          tunnel: [w435 w447] -> w428
          frame False {
            # "When Size is clicked for the second time"
            n154 = To Variant(anything=3) -> (Variant=w433:variant)
            n155 = Bundle By Name(cluster=T7 {"State"="", "Data"=variant} ("Dequeue Element"), "State"="Sort Tree Descending", "Data"=w433) -> (w438:T7)
            n156 = Bundle By Name(cluster=w444, "Sort Flag.Sort Size"=TRUE ("Trigger Sort")) -> (w443:T1)
            n157 = Build Array(w438) -> (w437:T7[])
            n158 = call "FileExplorerQueueDriver.vi"("Enqueue N Element"=w437, "error in (no error)"=w436, "Enum"=FileExplorerQueueOperations."Enqueue N") -> ("error out"=w435:errorcluster)  [unwired: 11 in, 1 out]
          }
          frame True {
            # "When Size is clicked once."
            n159 = To Variant(anything=3) -> (Variant=w445:variant)
            n160 = Bundle By Name(cluster=T7 {"State"="", "Data"=variant} ("Dequeue Element"), "State"="Sort Tree Ascending", "Data"=w445) -> (w450:T7)
            n161 = Bundle By Name(cluster=w456, "Sort Flag.Sort Size"=FALSE ("Trigger Sort")) -> (w455:T1)
            n162 = Build Array(w450) -> (w449:T7[])
            n163 = call "FileExplorerQueueDriver.vi"("Enqueue N Element"=w449, "error in (no error)"=w448, "Enum"=FileExplorerQueueOperations."Enqueue N") -> ("error out"=w447:errorcluster)  [unwired: 11 in, 1 out]
          }
        }
      }
      frame "/***COPY FILES***/" {
      }
      frame "Copy" {
        # "Copies the path of the selected files and creates a duplicate in the target path choosen from the file dialog."
        n164 = Unbundle By Name(w461) -> ("File Selection.Files Selected ?"=w460:bool)
        n165 = case shown="True" w460 {
          tunnel: [w469 w476] -> w465
          tunnel: [w468 w470] -> w464
          tunnel: w463 -> [w468 w474]
          tunnel: w461 -> [w469 w472]
          frame False {
            # "When copy button is pressed after without selecting any files"
            n166 = One Button Dialog(message="Select Files before Copy", button name ("OK")="Ok") -> ()  [unwired: 1 out]
          }
          frame True {
            # "When copy button is pressed after selecting files"
            n167 = call "File Dialog"("error in"=w474) -> ("selected path"=w475:path, "cancelled"=w471:bool, "error out"=w473:errorcluster)  [unwired: 11 in, 1 out]
            n168 = case shown="False" w471 {
              tunnel: [w479 w489] -> w476
              tunnel: w475 -> [_ w480]
              tunnel: [w477 w483] -> w470
              tunnel: w473 -> [w478 w487]
              tunnel: w472 -> [w479 w486]
              frame True {
                # "When cancel option of the file dialog is pressed."
                n169 = call <vilib>:"Clear Errors.vi"("error in (no error)"=w478) -> ("error out"=w477:errorcluster)  [unwired: 5 in, 1 out]
              }
              frame False {
                # "When folder path is selected using File Dialog."
                n170 = Unbundle By Name(w486) -> ("Copied File Path array"=w490:path[])
                n171 = for {
                  tunnel: w480 -> [w492]
                  shift-right: [w497] -> w484
                  shift-left: w487 -> [w494]
                  tunnel: w490 -> [w493] mode=indexing
                  tunnel: [w495] -> w482
                  # "Iterates the path of the selected files"
                  n172 = Strip Path(path=w493) -> (stripped path=w496:path)  [unwired: 1 out]
                  n173 = Equal?(x=w496, y=w492) -> (x = y?=w491:bool)
                  n174 = case shown="False" w491 {
                    tunnel: w494 -> [w501 w507]
                    tunnel: [w501 w506] -> w497
                    tunnel: w492 -> [_ w505]
                    tunnel: w493 -> [_ w504]
                    tunnel: [T7[] [] ("Enqueue N Element") T7[] [{"State"="Check New Folder", "Data"=variant}] ("Enqueue N Element")] -> w495
                    frame True {
                      # "When the selected file already exists in that folder"
                      n175 = One Button Dialog(message="File already exists ", button name ("OK")="OK") -> ()  [unwired: 1 out]
                    }
                    frame False {
                      # "When the selected file already does not exists in that folder"
                      n176 = Copy(8:w507, 9:TRUE ("overwrite (F)"), 10:w505, 11:w504) -> (0:w506:errorcluster)  [unwired: 1 in, 2 out]
                    }
                  }
                }
                n177 = Strip Path(path=w480) -> (stripped path=w481:path, name=w488:string)
                n178 = Bundle By Name(cluster=w486, "Paths.New Folder Dialog"=w481, "Copy file Folder"=w488, "New Folder Tag"=w480) -> (w489:T1)
                n179 = call "FileExplorerQueueDriver.vi"("Enqueue N Element"=w482, "error in (no error)"=w484, "Enum"=FileExplorerQueueOperations."Enqueue N") -> ("error out"=w483:errorcluster)  [unwired: 11 in, 1 out]
              }
            }
          }
        }
      }
      frame "Check New Folder" {
        # "When the selected file is tried to copied in a new folder, that particular new folder is populated in the tree."
        n180 = Unbundle By Name(w510) -> ("Copy file Folder"=w511:string)
        n181 = property on="Tree" class="Tree (strict)"(error in=w513) -> (error out=w512:errorcluster, "All Tags"=w514:string[])  [unwired: 1 in, 1 out]
        n182 = for {
          shift-right: [w531] -> w516
          shift-left: w512 -> [w531]
          tunnel: w514 -> [w534] mode=indexing
          tunnel: w511 -> [w535]
          shift-right: [w527] -> w509
          shift-left: w510 -> [w530]
          # "Iterates to check there exists a folder already with the name of newly create folder."
          n183 = String To Path(string=w534) -> (path=w533:path)
          n184 = Strip Path(path=w533) -> (name=w532:string)  [unwired: 1 out]
          n185 = Unbundle By Name(w530) -> ("New Folder"=w528:bool)
          n186 = Not Equal?(x=w535, y=w532) -> (x != y?=w529:bool)
          n187 = And(x=w528, y=w529) -> (x .and. y?=w526:bool)
          n188 = Bundle By Name(cluster=w530, "New Folder"=w526) -> (w527:T1)
        }
        n189 = Unbundle By Name(w509) -> ("New Folder"=w508:bool)
        n190 = case shown="False" w508 {
          tunnel: w516 -> [w519 w524]
          tunnel: [w518 w523] -> w515
          frame False {
            # "When new folder is not created"
            n191 = call "FileExplorerQueueDriver.vi"("Enqueue Element"=T7 {"State"="Populate Copied Files", "Data"=variant}, "error in (no error)"=w519, "Enum"=FileExplorerQueueOperations."Enqueue") -> ("error out"=w518:errorcluster)  [unwired: 11 in, 1 out]
          }
          frame True {
            # "When new folder is created"
            n192 = call "FileExplorerQueueDriver.vi"("Enqueue Element"=T7 {"State"="Populate New Folder", "Data"=variant}, "error in (no error)"=w524, "Enum"=FileExplorerQueueOperations."Enqueue") -> ("error out"=w523:errorcluster)  [unwired: 11 in, 1 out]
          }
        }
      }
      frame "Populate New Folder" {
        # "When the selected file is tried to copied in a new folder, that particular new folder is populated in the tree."
        n193 = Unbundle By Name(w546) -> ("New Folder Tag"=w536:path, "Copy file Folder"=w538:string, "Paths.New Folder Dialog"=w537:path)
        n194 = property on="Tree" class="Tree (strict)"(error in=w540) -> (error out=w539:errorcluster, "All Tags"=w541:string[])  [unwired: 1 in, 1 out]
        n195 = for {
          shift-right: [w565] -> w544
          shift-left: w539 -> [w564]
          tunnel: w541 -> [w561] mode=indexing
          tunnel: w538 -> [w562]
          tunnel: w537 -> [w563]
          tunnel: w536 -> [w560]
          # "Iterates to check there exists a folder already with the name of newly create folder."
          n196 = String To Path(string=w561) -> (path=w559:path)
          n197 = Strip Path(path=w559) -> (name=w558:string)  [unwired: 1 out]
          n198 = File/Directory Info(path=w563, error in=w564) -> (size=w553:i64, last mod=w555:timestamp, error out=w548:errorcluster)  [unwired: 4 out]
          n199 = Number To Fractional String(number=w553, precision (6)=i16 0) -> (F-format string=w552:string)  [unwired: 2 in]
          n200 = Get Date/Time String(seconds (now)=w555) -> (date string=w554:string)  [unwired: 2 in, 1 out]
          n201 = Strip Path(path=w563) -> (name=w557:string)  [unwired: 1 out]
          n202 = Equal?(x=w557, y=w558) -> (x = y?=w556:bool)
          n203 = Build Array(w554, "Folder" ("element"), w552) -> (w549:string[])
          n204 = case shown="True" w556 {
            tunnel: w548 -> [w566 w577]
            tunnel: [w566 w575] -> w565
            tunnel: w562 -> [_ w573]
            tunnel: w549 -> [_ w572]
            tunnel: w560 -> [_ w571]
            frame False {
              # "when new folder is not created."
            }
            frame True {
              # "Populates the newly created folder"
              n205 = Strip Path(path=w571) -> (stripped path=w568:path)  [unwired: 1 out]
              n206 = Path To String(path=w571) -> (string=w570:string)
              n207 = Path To String(path=w568) -> (string=w569:string)
              n208 = invoke on="Tree" class="Tree (strict)" method="Edit Tree Items.Add Item"(error in=w577, "Parent Tag"=w569, "Left Cell"=w573, "Child Text"=w572, "Child Tag"=w570, "Child Only?"=FALSE) -> (error out=w576:errorcluster)  [unwired: 3 in, 8 out]
              n209 = property on="Tree" class="Tree (strict)"(error in=w576, "Active Item Tag"=w570, "Glyph"=37 ("Active Item:Symbol Index")) -> (error out=w575:errorcluster)  [unwired: 1 in, 1 out]
            }
          }
        }
        n210 = call "FileExplorerQueueDriver.vi"("Enqueue Element"=T7 {"State"="Populate Copied Files", "Data"=variant}, "error in (no error)"=w544, "Enum"=FileExplorerQueueOperations."Enqueue") -> ("error out"=w543:errorcluster)  [unwired: 11 in, 1 out]
      }
      frame "Selected Files" {
        # "Selected tree item is check whether a file or folder and when it is a file, selected file is added to an array."
        n211 = Variant To Data(error in=w590, type="" ("Tag"), Variant=w589) -> (data=w579:string, error out=w585:errorcluster)
        n212 = First Call?() -> (First Call?: T/F=w578:bool)
        n213 = case shown="True" w578 {
          tunnel: w587 -> [w591 w594]
          tunnel: [w591 w593] -> w580
          tunnel: w579 -> [_ w592]
          frame False {
          }
          frame True {
            n214 = Bundle By Name(cluster=w594, "File Selection.First Selection"=w592) -> (w593:T1)
          }
        }
        n215 = property on="Tree" class="Tree (strict)"(error in=w585, "Active Item Tag"=w579) -> (error out=w583:errorcluster, "Child-Only?"=w582:bool)  [unwired: 1 in, 1 out]
        n216 = case shown="True" w582 {
          selector: w582 -> [_ w607]
          tunnel: w580 -> [w596 w606]
          tunnel: [w596 w608] -> w586
          tunnel: [w595 w604] -> w584
          tunnel: w583 -> [w595 w605]
          tunnel: w579 -> [_ w600]
          frame False {
            # "When the selected files are not a child-only file"
          }
          frame True {
            # "When the selected files are child-only files."
            n217 = Unbundle By Name(w606) -> ("File Selection.First Selection"=w603:string)
            n218 = String To Path(string=w600) -> (path=w601:path)
            n219 = String To Path(string=w603) -> (path=w602:path)
            n220 = Strip Path(path=w602) -> (stripped path=w599:path)  [unwired: 1 out]
            n221 = Strip Path(path=w601) -> (stripped path=w598:path)  [unwired: 1 out]
            n222 = Equal?(x=w599, y=w598) -> (x = y?=w597:bool)
            n223 = case shown="True" w597 {
              tunnel: [w610 w619] -> w608
              tunnel: w607 -> [_ w615]
              tunnel: w600 -> [_ w614]
              tunnel: w606 -> [w610 w612]
              tunnel: w605 -> [w609 w611]
              tunnel: [w609 w611] -> w604
              frame False {
              }
              frame True {
                n224 = Unbundle By Name(w612) -> ("File Selection.Selected file array"=w620:string[], "Copied File Path array"=w617:path[])
                n225 = Build Array (concatenate)(w620, w614) -> (w618:string[])
                n226 = String To Path(string=w614) -> (path=w613:path)
                n227 = Build Array (concatenate)(w617, w613) -> (w616:path[])
                n228 = Bundle By Name(cluster=w612, "File Selection.Selected file array"=w618, "Copied File Path array"=w616, "File Selection.Files Selected ?"=w615) -> (w619:T1)
              }
            }
          }
        }
      }
      frame "Populate Copied Files" {
        # "Added files in the array is then populated in the tree with its corresponding folder."
        n229 = Unbundle By Name(w624) -> ("New Folder Tag"=w625:path, "File Selection.Selected file array"=w633:string[], "Copy file Folder"=w632:string, "Copied File Path array"=w629:path[])
        n230 = property on="Tree" class="Tree (strict)"(error in=w628) -> (error out=w627:errorcluster, "All Tags"=w626:string[])  [unwired: 1 in, 1 out]
        n231 = for {
          tunnel: w633 -> [w645]
          tunnel: w632 -> [w643]
          shift-right: [w647] -> w636
          shift-left: w627 -> [w646]
          tunnel: w629 -> [w642]
          tunnel: w626 -> [w641] mode=indexing
          tunnel: w625 -> [w638]
          tunnel: w624 -> [w637]
          tunnel: [w637] -> w623
          # "Iterates to check the choosen folder already exists in the tree."
          n232 = String To Path(string=w641) -> (path=w640:path)
          n233 = Strip Path(path=w640) -> (name=w639:string)  [unwired: 1 out]
          n234 = Equal?(x=w643, y=w639) -> (x = y?=w644:bool)
          n235 = case shown="True" w644 {
            tunnel: [w648 w653] -> w647
            tunnel: w646 -> [w648 w652]
            tunnel: w645 -> [_ w651]
            tunnel: w642 -> [_ w650]
            tunnel: w638 -> [_ w649]
            frame False {
              # "When the folder path choosen from the file dialog is parallel to the input file path."
            }
            frame True {
              # "When the folder path choosen from the file dialog is parallel to the input file path."
              n236 = for {
                tunnel: w651 -> [w659] mode=indexing
                shift-right: [w676] -> w653
                shift-left: w652 -> [w666]
                tunnel: w650 -> [w665] mode=indexing
                tunnel: w649 -> [w656]
                # "Iterates to populate the copied  files in the tree"
                n237 = File/Directory Info(path=w665, error in=w666) -> (path out=w671:path, size=w674:i64, last mod=w675:timestamp, error out=w672:errorcluster)  [unwired: 3 out]
                n238 = Path To String(path=w656) -> (string=w655:string)
                n239 = Number To Fractional String(number=w674, precision (6)=i16 0) -> (F-format string=w661:string)  [unwired: 2 in]
                n240 = Get Date/Time String(seconds (now)=w675) -> (date string=w662:string)  [unwired: 2 in, 1 out]
                n241 = Get Type and Creator(4:w672, 7:w671) -> (0:w664:errorcluster, 2:w668:string)  [unwired: 2 out]
                n242 = Not Equal?(x=w668, y="????") -> (x != y?=w669:bool)
                n243 = String To Path(string=w659) -> (path=w658:path)
                n244 = Select(t=w668, s=w669, f="File") -> (s? t:f=w663:string)
                n245 = Strip Path(path=w658) -> (name=w657:string)  [unwired: 1 out]
                n246 = Build Array(w662, w663, w661) -> (w660:string[])
                n247 = invoke on="Tree" class="Tree (strict)" method="Edit Tree Items.Add Item"(error in=w664, "Parent Tag"=w655, "Left Cell"=w657, "Child Text"=w660, "Child Tag"=w659, "Child Only?"=FALSE) -> (error out=w676:errorcluster)  [unwired: 3 in, 8 out]
              }
            }
          }
        }
        n248 = Bundle By Name(cluster=w623, "File Selection.Selected file array"=string[] [] ("Selected file array"), "Copied File Path array"=path[] []) -> (w635:T1)
        n249 = One Button Dialog(message="Successfully Copied !!", button name ("OK")="OK") -> ()  [unwired: 1 out]
      }
      frame "/***EXPAND COLAPSE TREE***/" {
      }
      frame "Expand or ColapseTree" {
        # "Expands or collapses the tree when pressed."
        n250 = Unbundle By Name(w683) -> ("Paths.File Path"=w682:path)
        n251 = call <vilib>:"Is Path and Not Empty.vi"("path"=w682) -> ("Is Path and Not Empty?"=w680:bool)  [unwired: 4 in]
        n252 = Variant To Data(error in=w690, type=TRUE, Variant=w688) -> (data=w684:bool, error out=w689:errorcluster)
        n253 = case shown="True" w680 {
          tunnel: w689 -> [w693 w698]
          tunnel: [w693 w695] -> w685
          tunnel: w684 -> [_ w697]
          tunnel: w683 -> [w694 w696]
          tunnel: [w694 w696] -> w681
          frame False {
            # "When the tree us not populated and tried to expand or collapse"
            n254 = One Button Dialog(message="Populate Tree to Expand/Collapse", button name ("OK")="OK") -> ()  [unwired: 1 out]
          }
          frame True {
            # "When the path is valid and not empty."
            n255 = invoke on="Tree" class="Tree (strict)" method="Open/Close.Open/Close All"(error in=w698, "Open"=w697) -> (error out=w695:errorcluster)  [unwired: 2 in, 3 out]
          }
        }
      }
      frame "/***SEARCH FILE ***/" {
      }
      frame "Search Folder" {
        # "Opens the searched file in the tree when it is found."
        n256 = Variant To Data(error in=w715, type="", Variant=w714) -> (data=w706:string, error out=w709:errorcluster)
        n257 = property on="Tree" class="Tree (strict)"(error in=w709) -> (error out=w708:errorcluster, "All Tags"=w707:string[])  [unwired: 1 in, 1 out]
        n258 = for {
          shift-right: [w720] -> w710
          shift-left: w711 -> [w721]
          shift-right: [w718] -> w703
          shift-left: w708 -> [w719]
          tunnel: w707 -> [w717] mode=indexing
          tunnel: w706 -> [w723]
          # "Iterates to search for folder"
          n259 = String To Path(string=w717) -> (path=w724:path)
          n260 = Strip Path(path=w724) -> (name=w722:string)  [unwired: 1 out]
          n261 = Equal?(x=w723, y=w722) -> (x = y?=w716:bool)
          n262 = case shown="True" w716 {
            tunnel: w721 -> [w726 w728]
            tunnel: [w726 w732] -> w720
            tunnel: w719 -> [w725 w731]
            tunnel: [w725 w731] -> w718
            tunnel: w717 -> [_ w730]
            frame False {
              # "When searched folder is found"
            }
            frame True {
              # "When the searched folder is found"
              n263 = Unbundle By Name(w728) -> ("Searched Folder Tag"=w727:string[])
              n264 = Build Array (concatenate)(w727, w730) -> (w729:string[])
              n265 = Bundle By Name(cluster=w728, "Searched Folder Tag"=w729) -> (w732:T1)
            }
          }
        }
        n266 = call "FileExplorerQueueDriver.vi"("Enqueue Element"=T7 {"State"="Expand Searced File", "Data"=variant}, "error in (no error)"=w703, "Enum"=FileExplorerQueueOperations."Enqueue") -> ("error out"=w702:errorcluster)  [unwired: 11 in, 1 out]
      }
      frame "Expand Searced File" {
        # "Opens the searched file in the tree when it is found."
        n267 = Unbundle By Name(w735) -> ("Searched Folder Tag"=w733:string[])
        n268 = Empty Array?(array=w733) -> (empty?=w734:bool)
        n269 = case shown="False" w734 {
          tunnel: w735 -> [w743 w749]
          tunnel: [w743 w748] -> w738
          tunnel: [w744 w747] -> w737
          tunnel: w736 -> [w744 w746]
          tunnel: w733 -> [_ w745]
          frame True {
            # "When search bar is empty or not found"
            n270 = local write "Search Bar"("" ("Search Bar")) -> ()
            n271 = One Button Dialog(message="Folder Not Found", button name ("OK")="OK") -> ()  [unwired: 1 out]
          }
          frame False {
            # "When search bar is valid and not empty"
            n272 = for {
              tunnel: w745 -> [w750] mode=indexing
              shift-right: [w757] -> w748
              shift-left: w749 -> [w758]
              shift-right: [w756] -> w747
              shift-left: w746 -> [w755]
              n273 = property on="Tree" class="Tree (strict)"(error in=w755, "Active Item Tag"=w750) -> (error out=w754:errorcluster)  [unwired: 1 in, 1 out]
              n274 = invoke on="Tree" class="Tree (strict)" method="Open/Close.Item"(error in=w754, "tag"=w750, "Open"=TRUE ("Open?")) -> (error out=w753:errorcluster)  [unwired: 2 in, 4 out]
              n275 = Bundle By Name(cluster=w758, "Searched Folder Tag"=string[] []) -> (w757:T1)
              n276 = invoke on="Tree" class="Tree (strict)" method="Open/Close.Ensure Visible"(error in=w753, "tag"=w750) -> (error out=w756:errorcluster)  [unwired: 2 in, 3 out]
            }
          }
        }
      }
      frame "/***FRONT PANEL UPDATE***/" {
      }
      frame "FP Update" {
        # "Updates the front panel indicators."
        n277 = Unbundle By Name(w764) -> ("Report details.Report String"=→"Report String":string)
      }
      frame "/***ERROR***/" {
      }
      frame "Error" {
        # "When any error occurs, this state popups the error and state from where the error has occured."
        n278 = Unbundle By Name(w780) -> ("status"=w776:bool, "code"=w775:i32)
        n279 = call <vilib>:"Clear Errors.vi"("error in (no error)"=w780) -> ("error out"=w779:errorcluster)  [unwired: 5 in, 1 out]
        n280 = Format Into String(format string="Erro occured at State : %s \nError Status : %s\nError Code : %d", initial string="", error in=w779, w777, w776, w775) -> (resulting string=w772:string, error out=w778:errorcluster)
        n281 = Two Button Dialog(message=w772, 1:"Exit" ("F button name (\"Cancel\")"), 2:"Continue" ("T button name (\"OK\")")) -> (T button?=w769:bool)
        n282 = Unbundle By Name(w785) -> ("user event ref"=w784:refnum<user-event>)
        n283 = case shown="False" w769 {
          tunnel: [w787 w794] -> w786
          tunnel: w778 -> [w787 w791]
          tunnel: w784 -> [w788 w790]
          tunnel: [w788 w789] -> w782
          frame True {
          }
          frame False {
            # "When user clicks Exit after an error occurs, and when exit is presed VI is aborted"
            n284 = call "FileExplorerQueueDriver.vi"("Enqueue Element"=T7 {"State"="Exit", "Data"=variant}, "error in (no error)"=w791, "Enum"=FileExplorerQueueOperations."Enqueue") -> ("error out"=w795:errorcluster)  [unwired: 11 in, 1 out]
            n285 = Generate User Event(user event=w790, event data cluster=TRUE ("event data"), error in=w795) -> (user event out=w789:refnum<user-event>, error out=w794:errorcluster)  [unwired: 1 in]
          }
        }
        n286 = Bundle By Name(cluster=w785, "user event ref"=w782) -> (w783:T1)
      }
      frame "Exit" {
        # "Exits the consumer loop."
        n287 = call "FileExplorerQueueDriver.vi"("error in (no error)"=w801, "Enum"=FileExplorerQueueOperations."Flush") -> ("error out"=w800:errorcluster)  [unwired: 12 in, 1 out]
        n288 = call "FileExplorerQueueDriver.vi"("error in (no error)"=w800, "Enum"=FileExplorerQueueOperations."Close") -> ("error out"=w799:errorcluster)  [unwired: 12 in, 1 out]
      }
    }
  }
  n289 = while {
    shift-right: [w808] -> w16
    shift-left: w9 -> [w809]
    tunnel: w8 -> [w805]
    tunnel: [w804] -> w6
    stop <- w806 stop-if-true
    # "Producer Loop."
    n290 = event shown="[2] \"Tree\": Mouse Down" {
      selector: w805 -> [_ _ _ _ _ _ _ _]
      dyn-events: [_ _ _ _ _ _ _ _] -> w804
      timeout: 50 -> [_ _ _ _ _ _ _ _]
      tunnel: w809 -> [w811 w817 w838 w844 w850 w854 w859 w869]
      tunnel: [w811 w816 w837 w843 w849 w854 w858 w868] -> w808
      tunnel: [FALSE FALSE ("Stop") FALSE ("Stop") FALSE ("Stop") w853 w855 FALSE ("Stop") FALSE ("Stop")] -> w806
      event Timeout {
        # "Timeout is executed when no other event is triggered."
        n291 = event-data() -> ()  [unwired: 1 in, 1 out]
      }
      event "Top Level Folder Path": Value Change {
        # "This event is triggered when there is a value change in the folder path control."
        n292 = event-data() -> ("NewVal"=w815:path)  [unwired: 1 in]
        n293 = To Variant(anything=w815) -> (Variant=w814:variant)
        n294 = Bundle By Name(cluster=T7 {"State"="", "Data"=variant} ("Dequeue Element"), "State"="Get Path", "Data"=w814) -> (w812:T7)
        n295 = call "FileExplorerQueueDriver.vi"("Enqueue Element"=w812, "error in (no error)"=w817, "Enum"=FileExplorerQueueOperations."Enqueue") -> ("error out"=w816:errorcluster)  [unwired: 11 in, 1 out]
      }
      event "Tree": Mouse Down {
        # "Thiis event is triggered when the mouse is pressed down on any tree item."
        n296 = event-data() -> ("Coords"=w835:T9)  [unwired: 1 in]
        n297 = invoke on="Tree" class="Tree (strict)" method="Point To Row Column"(error in=w838, "Point"=w835) -> (error out=w836:errorcluster, "Tag"=w829:string, "Col"=w834:i32, "InGlyph"=w824:bool)  [unwired: 6 in, 4 out]
        n298 = Number To Fractional String(number=w834, precision (6)=i16 0) -> (F-format string=w828:string)  [unwired: 2 in]
        n299 = Select(t="InSymbolTrue" ("F-format string"), s=w824, f="InSymbolFalse") -> (s? t:f=w821:string)
        n300 = Build Array(w829, w828, w821) -> (w827:string[])
        n301 = To Variant(anything=w827) -> (Variant=w830:variant)
        n302 = Bundle By Name(cluster=T7 {"State"="", "Data"=variant} ("Dequeue Element"), "State"="Trigger Sort", "Data"=w830) -> (w825:T7)
        n303 = call "FileExplorerQueueDriver.vi"("Enqueue Element"=w825, "error in (no error)"=w836, "Enum"=FileExplorerQueueOperations."Enqueue") -> ("error out"=w837:errorcluster)  [unwired: 11 in, 1 out]
      }
      event "Copy": Value Change {
        # "Thi event is triggered when there is a value change in the copy boolean."
        n304 = event-data() -> ("NewVal"=w842:bool)  [unwired: 1 in]
        n305 = To Variant(anything=w842) -> (Variant=w848:variant)
        n306 = Bundle By Name(cluster=T7 {"State"="", "Data"=variant} ("Dequeue Element"), "State"="Copy", "Data"=w848) -> (w840:T7)
        n307 = call "FileExplorerQueueDriver.vi"("Enqueue Element"=w840, "error in (no error)"=w844, "Enum"=FileExplorerQueueOperations."Enqueue") -> ("error out"=w843:errorcluster)  [unwired: 11 in, 1 out]
      }
      event Panel Close? {
        w853 = TRUE ("Discard?")
        # "This event is triggered when the front panel is closed."
        n308 = event-data() -> ()  [unwired: 1 in, 1 out]
        n309 = call "FileExplorerQueueDriver.vi"("Enqueue Element"=T7 {"State"="Exit", "Data"=variant}, "error in (no error)"=w850, "Enum"=FileExplorerQueueOperations."Enqueue") -> ("error out"=w849:errorcluster)  [unwired: 11 in, 1 out]
        n310 = event-data("Discard?"=w853) -> ()  [unwired: 1 in, 1 out]
      }
      event User Event {
        # "This event stops this producer loop when stop user event is generated in the consumer loop."
        n311 = event-data() -> ("Stop"=w855:bool)  [unwired: 1 in]
      }
      event "Expand / Colapse": Value Change {
        # "Thi event is triggered when there is a value change in the collapse boolean."
        n312 = event-data() -> ("NewVal"=w863:bool)  [unwired: 1 in]
        n313 = To Variant(anything=w863) -> (Variant=w862:variant)
        n314 = Bundle By Name(cluster=T7 {"State"="", "Data"=variant} ("Dequeue Element"), "State"="Expand or ColapseTree", "Data"=w862) -> (w856:T7)
        n315 = call "FileExplorerQueueDriver.vi"("Enqueue Element"=w856, "error in (no error)"=w859, "Enum"=FileExplorerQueueOperations."Enqueue") -> ("error out"=w858:errorcluster)  [unwired: 11 in, 1 out]
      }
      event "Search Bar": Value Change {
        # "Thi event is triggered when there is a value change in the search bar- string control."
        n316 = event-data() -> ("NewVal"=w867:string)  [unwired: 1 in]
        n317 = To Variant(anything=w867) -> (Variant=w866:variant)
        n318 = Bundle By Name(cluster=T7 {"State"="", "Data"=variant} ("Dequeue Element"), "State"="Search Folder", "Data"=w866) -> (w865:T7)
        n319 = call "FileExplorerQueueDriver.vi"("Enqueue Element"=w865, "error in (no error)"=w869, "Enum"=FileExplorerQueueOperations."Enqueue") -> ("error out"=w868:errorcluster)  [unwired: 11 in, 1 out]
      }
    }
  }
  n320 = Unregister For Events(event registration refnum=w6, error in=w16) -> (error out=w7:errorcluster)
  n321 = Destroy User Event(user event=w3, error in=w7) -> (error out=w5:errorcluster)
  n322 = Merge Errors(w5, w17) -> (→"error out":errorcluster)
